vi "Dashboard Main.vi"() -> ()   [LabVIEW 2023]
uses:
  <vilib>/Utility/miscctls.llb/LVRectTypeDef.ctl
  <vilib>/event_ctls.llb/eventvkey.ctl
  <vilib>/Rock Robotics/WPI/DriverStation/WPI_DriverStationAllianceInfo.ctl
  b1c29fd4-b69e-4c47-bd92-218700034153.vi
  cd51690b-7cbe-44fb-a5f0-3232adb0ed53.vi
  a4e8d5d1-2ec3-4e81-be0b-60391cc68073.vi
  1b78be80-bab2-445d-a3e8-82f142a16380.vi
  9e807339-2903-4f51-8fcc-64b6a9381567.vi
  e75f20ac-3dfa-4544-8614-4803d6d17fbb.vi
  273c17a0-a238-4f2a-a55a-7e29d73850ff.vi
  87bdd142-1820-4e26-8582-f713a5f3da40.vi
  b8451b18-7b16-4e07-a196-a1bebf8ce026.vi
  5d307e9f-edd0-4132-a387-09c5916d43b1.vi
  0137daef-9682-45ba-80b9-2d4fda8852b8.vi
  f6a63fab-964b-4051-8314-d4414a0a258c.vi
  90e0fe9d-42b1-4a72-a6c8-4b9d9b3a5a2a.vi
  f15e925d-3118-43e3-bf67-a1272bbf81dd.vi
  394886aa-4cdd-4740-8681-89e3e438764a.vi
  77a42c1f-99bf-4bb6-8218-45b49017f7dc.vi
  5abae45b-ab2b-4816-ba0c-2a0b218f6531.vi
  31f70c1d-3051-4c77-9544-a691198ba614.vi
  f63f5451-5db6-487e-bc86-5cb81e92b132.vi
  81d0db6a-d68a-45c3-b3b1-458879412541.vi
  c235c188-eb56-46fb-93d3-e8acf396af31.vi
  115ba94a-0b26-47fa-ae73-5ec5bd9e502a.vi
  2422668c-951b-48e5-9bda-0f59c56d9c0d.vi
  7776664e-4af7-4b3d-b288-2266642a045e.vi
  6004ed5d-dfc4-4dad-95c1-8e371ea2b9cd.vi
  321ce103-7778-4bb1-9ecc-75a76fef05e9.vi
  d30e88cc-5e2b-4867-b271-53fc6d5cd4d7.vi
  fde90579-e212-4b8a-8145-a17c3e40bcbd.vi
  6c63589b-432e-4f9c-bacb-2063ed7bd576.vi
  b7dcf304-99f6-4f78-9d14-19aa8d9ea562.vi
  e8b3bb93-ba91-445b-94c6-9e998421f827.vi
  0480a820-69ef-45e6-a9f4-d7ff60c89e45.vi
  1c99237e-ea3d-4ecf-b7c2-61034db3ecd2.vi
  0a8fe2ab-d060-4915-a9b5-d8978247e2b6.vi
  b1c29fd4-b69e-4c47-bd92-218700034153.vi/77c742ae-e671-49bb-a825-a6e8cebc9f63.vi
  cd51690b-7cbe-44fb-a5f0-3232adb0ed53.vi/77c742ae-e671-49bb-a825-a6e8cebc9f63.vi
  a4e8d5d1-2ec3-4e81-be0b-60391cc68073.vi/77c742ae-e671-49bb-a825-a6e8cebc9f63.vi
  1b78be80-bab2-445d-a3e8-82f142a16380.vi/77c742ae-e671-49bb-a825-a6e8cebc9f63.vi
  9e807339-2903-4f51-8fcc-64b6a9381567.vi/77c742ae-e671-49bb-a825-a6e8cebc9f63.vi
  e75f20ac-3dfa-4544-8614-4803d6d17fbb.vi/77c742ae-e671-49bb-a825-a6e8cebc9f63.vi
  0137daef-9682-45ba-80b9-2d4fda8852b8.vi/77c742ae-e671-49bb-a825-a6e8cebc9f63.vi
  f6a63fab-964b-4051-8314-d4414a0a258c.vi/77c742ae-e671-49bb-a825-a6e8cebc9f63.vi
  90e0fe9d-42b1-4a72-a6c8-4b9d9b3a5a2a.vi/77c742ae-e671-49bb-a825-a6e8cebc9f63.vi
  f15e925d-3118-43e3-bf67-a1272bbf81dd.vi/77c742ae-e671-49bb-a825-a6e8cebc9f63.vi
  394886aa-4cdd-4740-8681-89e3e438764a.vi/77c742ae-e671-49bb-a825-a6e8cebc9f63.vi
  77a42c1f-99bf-4bb6-8218-45b49017f7dc.vi/77c742ae-e671-49bb-a825-a6e8cebc9f63.vi
  5abae45b-ab2b-4816-ba0c-2a0b218f6531.vi/77c742ae-e671-49bb-a825-a6e8cebc9f63.vi
  31f70c1d-3051-4c77-9544-a691198ba614.vi/77c742ae-e671-49bb-a825-a6e8cebc9f63.vi
  f63f5451-5db6-487e-bc86-5cb81e92b132.vi/77c742ae-e671-49bb-a825-a6e8cebc9f63.vi
  81d0db6a-d68a-45c3-b3b1-458879412541.vi/77c742ae-e671-49bb-a825-a6e8cebc9f63.vi
  c235c188-eb56-46fb-93d3-e8acf396af31.vi/77c742ae-e671-49bb-a825-a6e8cebc9f63.vi
  115ba94a-0b26-47fa-ae73-5ec5bd9e502a.vi/77c742ae-e671-49bb-a825-a6e8cebc9f63.vi
  2422668c-951b-48e5-9bda-0f59c56d9c0d.vi/77c742ae-e671-49bb-a825-a6e8cebc9f63.vi
  7776664e-4af7-4b3d-b288-2266642a045e.vi/77c742ae-e671-49bb-a825-a6e8cebc9f63.vi
  6004ed5d-dfc4-4dad-95c1-8e371ea2b9cd.vi/77c742ae-e671-49bb-a825-a6e8cebc9f63.vi
  321ce103-7778-4bb1-9ecc-75a76fef05e9.vi/77c742ae-e671-49bb-a825-a6e8cebc9f63.vi
  d30e88cc-5e2b-4867-b271-53fc6d5cd4d7.vi/77c742ae-e671-49bb-a825-a6e8cebc9f63.vi
  fde90579-e212-4b8a-8145-a17c3e40bcbd.vi/77c742ae-e671-49bb-a825-a6e8cebc9f63.vi
  6c63589b-432e-4f9c-bacb-2063ed7bd576.vi/77c742ae-e671-49bb-a825-a6e8cebc9f63.vi
  b7dcf304-99f6-4f78-9d14-19aa8d9ea562.vi/77c742ae-e671-49bb-a825-a6e8cebc9f63.vi
  e8b3bb93-ba91-445b-94c6-9e998421f827.vi/77c742ae-e671-49bb-a825-a6e8cebc9f63.vi
  0480a820-69ef-45e6-a9f4-d7ff60c89e45.vi/77c742ae-e671-49bb-a825-a6e8cebc9f63.vi
  1c99237e-ea3d-4ecf-b7c2-61034db3ecd2.vi/77c742ae-e671-49bb-a825-a6e8cebc9f63.vi
  0a8fe2ab-d060-4915-a9b5-d8978247e2b6.vi/77c742ae-e671-49bb-a825-a6e8cebc9f63.vi
  <vilib>/Utility/xml.llb/Read From XML File(array).vi
  <vilib>/Utility/xml.llb/Write to XML File(string).vi
  <vilib>/Rock Robotics/Network Tables/NT Read Number.vi
  <vilib>/Rock Robotics/Network Tables/NT Read Boolean.vi
  GlobalDashboard.vi
  <vilib>/Rock Robotics/Network Tables/NT Read String.vi
  <vilib>/Rock Robotics/Network Tables/NT Write Number.vi
  <vilib>/Rock Robotics/Network Tables/NT Read Numeric Array.vi
  <vilib>/Rock Robotics/Network Tables/NT Read String Array.vi
  <vilib>/Rock Robotics/Network Tables/NT Write Boolean.vi
  <vilib>/Rock Robotics/Network Tables/NT Read Boolean Array.vi
  <vilib>/Rock Robotics/Network Tables/NT Write String.vi
  <vilib>/Rock Robotics/Network Tables/NT Write Numeric Array.vi
  <vilib>/Rock Robotics/Network Tables/NT Write String Array.vi
  <vilib>/vision/NI_Vision_Development_Module.lvlib
panel:
  out "Indexer_Fault":bool
  out "Intake_Fault":bool
  out "Intake_Overheating":bool
  out "Elevator_Fault":bool
  out "Elevator_Overheating":bool
  in  "TCP":refnum<k5>
  in  "Dashboard Tab":T1(tab)=enum."Setup/Auto"
  in  "CheckList":i32(listbox)
  out "Heading_to_Target":dbl format="%.1f"
  out "Distance_to_Target":dbl format="%.1f"
  out "Robot_P":dbl format="%.1f"
  in  "Enable_Streaming_GUI":bool=TRUE
  out "Robot_Profile_GUI":string
  out "Auto_Playbook_GUI":string
  in  "Select Driver Profile":u16(ring) items=["N/A"]
  in  "Camera Name":string(combo)="limelight"
  in  "Camera Settings":T2={"Frame Rate"=20, "Compression"=60, "Size"=1, "DB Camera Config"=FALSE} {"Size" items=["640x480", "320x240", "160x120"]}
  in  "Select Autonomous Play":u16(ring) items=["N/A"]
  out "Master_Caution_GUI_0":bool caption="Mode_Butterfly"
  out "Robot_is_Autonomous_GUI_0":bool caption="Mode_Butterfly"
  out "Robot_Code_Version_GUI":string
  out "Auto_Suffix_GUI":string
  in  "Refresh_Auto_Play_List_GUI":bool
  in  "Auto_Delay_GUI":dbl format="%.1f"
  in  "Manual_Start_X":dbl min=0.0 max=700.0 format="%.1f"
  out "Robot_X":dbl format="%.1f"
  out "Robot_Y":dbl format="%.1f"
  in  "Manual_Start_Y":dbl min=0.0 max=400.0 format="%.1f"
  out "Robot_H_GUI":dbl format="%.1f"
  in  "Manual_Start_H":dbl min=0.0 max=360.0 format="%.1f"
  in  "Field Map":u16(ring) items=["N/A"]
  in  "Push_Robot_Start_GUI":bool
  in  "Export_Robot_Pose":bool
  in  "Clear_Robot_Pose_Display":bool
  in  "Dock_Dashboard":bool
  in  "Force_Human_Control_GUI":bool
  in  "Auto_Test_Mode_GUI":bool
  in  "Disable_Fusion_While_Autonomous":bool
  in  "Disable_Fusion_While_Disabled":bool=TRUE
  out "Robot Pose 1":cluster{dbl[], dbl[]}[](graph)
  out "Master_State_TRAP_Indicator":bool
  out "Master_State_CLIMB_Indicator":bool
  out "Master_State_AMP_Indicator":bool
  out "Help Graphic":T3(plugin-control)
  out "LL_Ret_Left":bool
  out "LL_Ret_Right":bool
  out "WA_Ret_Right":bool
  out "WA_Ret_Left":bool
  out "Swerve_Drive_Fault":bool
  out "State_Score":bool
  out "State_Shelf":bool
  out "Robot Pose 2":cluster{dbl[], dbl[]}[](graph)
  out "Master_State_SPEAKER_Indicator":bool
  out "Vision_Fault_GUI":bool
  out "Pressure_Leak_GUI":bool
  in  "Master_Safety_Override_1":bool
  in  "Manipulator_Help":bool
  in  "Driver_Help":bool
  out "No_Secondary_Camera":bool
  out "Swerve_Shifter_Failure":bool
  out "Electrical_Fault_GUI":bool
  out "Diverting_Power_GUI":bool
  out "CAN_Bus_Fault_GUI":bool
  out "IMU_Failure_GUI":bool
  out "Robot_is_Autonomous_GUI_1":bool caption="Mode_Butterfly"
  out "LL_Valid":bool caption="Mode_Butterfly"
  out "Auto_Error_GUI":bool
  in  "Clear_Errors_GUI":bool
  out "Swerve_Azimuth_Fault":bool
  out "Pressure_Transducer_GUI":dbl(slide) scale=0.0..115.0
  out "Pressure_Vent_GUI":bool
  out "Swerve_Overheating":bool
  out "Compressor_On_GUI":bool
  in  "Right":bool
  in  "Reticule":T4(ring)
  in  "Save":bool
  in  "Up":bool
  in  "Down":bool
  in  "Left":bool
  out "Master_Caution_GUI_1":bool caption="Mode_Butterfly"
  out "Battery_Critical_GUI":bool
  out "Battery_Voltage_GUI":dbl(slide) scale=11.0..13.0
  out "Field_Oriented_GUI":bool caption="Mode_Butterfly"
  out "Slow_Loop":bool
  out "Combined Camera Feed":T3(plugin-control)
  in  "Camera_Override_GUI":bool
  in  "Field_Oriented_Override_GUI":bool
  out "Pointed_at_Target":bool caption="Mode_Butterfly"
  in  "Auto_Targeting_Override":bool
  out "State_Hopper":bool
  out "Using_Auto_Targeting":bool caption="Mode_Butterfly"
  out "Swerve_Output_Loop_Time_GU":u32
  out "Swerve_3_Drive_Velocity":dbl format="%.1f"
  out "Swerve_3_Azimuth_Position":dbl format="%.1f"
  out "Swerve_3_Drive_Temperature":dbl
  out "Swerve_0_Drive_Temperature":dbl
  out "Camera Perf":string
  out "Control_Loop_Time_GUI":u32
  in  "Calibrate_Wheels_GUI":bool
  in  "Home_Wheels_GUI":bool
  out "Swerve_0_Azimuth_Position":dbl format="%.1f"
  out "Swerve_0_Drive_Velocity":dbl format="%.1f"
  out "Swerve_1_Drive_Velocity":dbl format="%.1f"
  out "Swerve_1_Azimuth_Position":dbl format="%.1f"
  out "Swerve_1_Drive_Temperature":dbl
  out "Swerve_2_Drive_Velocity":dbl format="%.1f"
  out "Swerve_2_Azimuth_Position":dbl format="%.1f"
  out "Swerve_2_Drive_Temperature":dbl
  in  "Arm_Calibrate_Wheels_GUI":bool
  out "Master_Caution_GUI_2":bool caption="Mode_Butterfly"
  in  "Actuator Testing":u16(ring) items=["N/A"]
  in  "Test_Actuator_Value_GUI":dbl step=0.1 format="%.2f"
  in  "Calibrate_Joysticks_GUI":bool
  in  "Arm_Calibrate_Joysticks":bool
  out "Robot_is_Autonomous_GUI_2":bool caption="Mode_Butterfly"
  in  "Test_Actuator_Period_GUI":dbl min=0.0 step=1.0 format="%.2f"
  out "Pose_Loop_Time_GUI":u32
  in  "Mute_Audible_Warnings":bool
  out "Combined Error String":string
  out "Swerve_0_Shifter_State":string
  out "Swerve_1_Shifter_State":string
  out "Swerve_3_Shifter_State":string
  out "Swerve_2_Shifter_State":string
  out "Swerve_Azimuth_Fault_Array":bool[](array[boolean])
  in  "Super_Test_Mode_GUI":bool
  out "Current_Driver_Profile_Setpoints_GUI":T5={"Strafe Deadband"=0.08, "Strafe Scaling"=2.0, "Strafe Maximum"=0.5, "Rotation Deadband"=0.15, "Rotation Scaling"=2.5, "Rotation Maximum"=0.5} {"Rotation Maximum" min=0.3 max=1.0 scale=0.3..1.0; "Rotation Scaling" min=1.0 max=4.0 scale=1.0..4.0; "Rotation Deadband" min=0.0 max=0.25 scale=0.0..0.25; "Strafe Maximum" min=0.3 max=1.0 scale=0.3..1.0; "Strafe Scaling" min=1.0 max=4.0 scale=1.0..4.0; "Strafe Deadband" min=0.0 max=0.25 scale=0.0..0.25}
  in  "New_Driver_Profile_Setpoints_GUI":T6={"Strafe Deadband"=0.08, "Strafe Scaling"=2.0, "Strafe Max"=0.5, "Rotate Deadband"=0.15, "Rotate Scaling"=2.5, "Rotate Max"=0.5} {"Rotate Max" min=0.3 max=1.0 format="%.2g"; "Rotate Scaling" min=1.0 max=4.0 format="%.2g"; "Rotate Deadband" min=0.0 max=0.25 format="%.2g"; "Strafe Max" min=0.3 max=1.0 format="%.2g"; "Strafe Scaling" min=1.0 max=4.0 format="%.2g"; "Strafe Deadband" min=0.0 max=0.25 format="%.2g"}
  in  "Apply_Driver_Profile_Setpoints_GUI":bool
  out "Current_Driver_Profile_GUI":string
  in  "Free_Tuning_Variable_GUI":dbl min=0.0 step=1.0 format="%.3f"
  out "Audible_Warnings_Enabled_GUI":bool
  out "Legal_Drivers_GUI":string[](array[string])
  out "Swerve_Shifter_Failure_Array":bool[](array[boolean])
  out "Swerve_Overheating_Array":bool[](array[boolean])
  out "Swerve_Drive_Fault_Array":bool[](array[boolean])
  out "NT Connection":bool
  out "Mode":T7(ring)=enum."Auto Disabled"
  out "Tree":string(tree)
  out "Background":bool
  # "2023 Dashboard v2.3-stable"
  # "Robot Profile"
  # "Robot X Position (in)"
  # "Robot Y Position (in)"
  # "Delay (s)"
  # "Robot Heading (deg)"
  # "Suffix"
  # "X (in)"
  # "Robot Pitch (deg)"
  # "Autonomous Playbook Entry"
  # "Auto Test\nMode"
  # "Force\nHuman"
  # "Y (in)"
  # "Target Distance (in)"
  # "Target Heading (deg)"
  # "H (deg)"
  # "Undock Dashboard"
  # "Yes Camera Streaming"
  # "Stop Fusion While Auto"
  # "Stop Fusion While Disabled"
  # "X"
  # "Y"
  # "MASTER\nSTATES"
  # "OVERRIDES"
  # "Camera Override"
  # "Robot-Oriented Drive Controls"
  # "Auto-Targeting Override"
  # "Disengage\nSafeties"
  # "11"
  # "13"
  # "0"
  # "120"
  # "Drivebase Subsytem"
  # "Driver Profile Selected"
  # "Loop Times"
  # "Module 1"
  # "Module 0"
  # "Control (ms)"
  # "Azimuth (deg)"
  # "Pose (ms)"
  # "Temp (C)"
  # "Drive Output (ms)"
  # "Velocity (ft/s)"
  # "Shifter State"
  # "Module 2"
  # "Module 3"
  # "Variable (bleh)"
  # "Disabled\nTest Mode"
  # "Azimuth (deg)"
  # "Temp (C)"
  # "Velocity (ft/s)"
  # "Shifter State"
  # "Calibrate Wheels"
  # "Period (s)"
  # "Calibrate Joysticks"
  # "Amplitude"
  # "0"
  # "0.25"
  # "1"
  # "4"
  # "0.3"
  # "1"
  # "0"
  # "0.25"
  # "1"
  # "4"
  # "0.3"
  # "1"
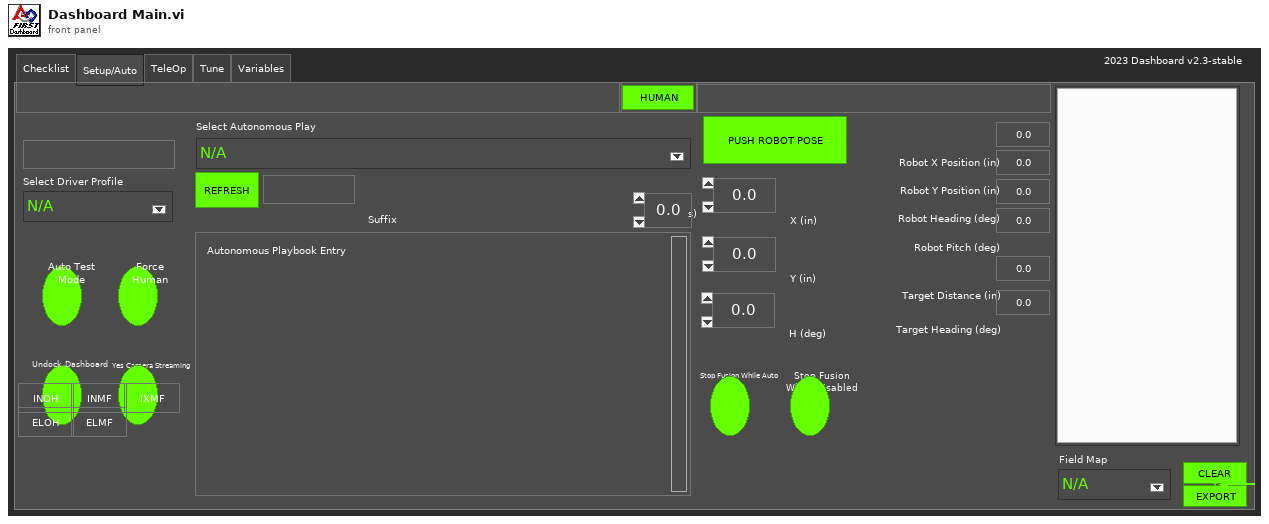
[diagram p1: front panel]
types:
  T1 = enum32{"Checklist", "Setup/Auto", "TeleOp", "Tune", "NT", "Test", "Commands", "Variables"}
  T2 = cluster{"Frame Rate":i32, "Compression":i32, "Size":u16, "DB Camera Config":bool}
  T3 = typedef "IMAQ Image.ctl" = refnum<image>
  T4 = enum16{"Wide Angle Left Reticule", "Wide Angle Right Reticule", "Lime Light Left Reticule", "Lime Light Right Reticule"}
  T5 = cluster{"Strafe Deadband":dbl, "Strafe Scaling":dbl, "Strafe Maximum":dbl, "Rotation Deadband":dbl, "Rotation Scaling":dbl, "Rotation Maximum":dbl}
  T6 = cluster{"Strafe Deadband":dbl, "Strafe Scaling":dbl, "Strafe Max":dbl, "Rotate Deadband":dbl, "Rotate Scaling":dbl, "Rotate Max":dbl}
  T7 = enum8{"Tele-Op Disabled", "Tele-Op Enabled", "Auto Disabled", "Auto Enabled", "Test Disabled", "Test Enabled", "Disconnected", "No Code", "E-Stop"}
  T8 = cluster{"Save Path":path, "Interval (s)":dbl, "Keep":i32}
  T9 = enum32{"Drive", "Camera", "Basic", "Custom", "Test", "Commands", "Checklist", "Variables"}
  T10 = cluster{"IDs":cluster{"RPC field ID":u16, "Unique ID":u16}, "String":string}
  T11 = typedef "Image Type" = u32
  T12 = typedef "WPI_DriverStationAllianceInfo.ctl" = enum16{"Red", "Blue", "Invalid"}
  T13 = enum8{"Enabled", "Disabled", "Disabled and Grayed Out"}
  T14 = cluster{"Error Strings":string, "Disable Counts":cluster{u16, u16}, "Rail Faults":cluster{u16, u16, u16}, "Robot IP":string, "DB Mode":u8, "Event Info":cluster{"Name":string, "Type":u8, "Number":u16, "Replay":u8}}
  T15 = cluster{"Storage":cluster{"Disk Free":u64, "RAM Block":u32, "RAM free":u32}, "CPU Utilization":cluster{"CPU % ISR":sgl, "CPU % Time Crit":sgl, "CPU % Timed Str":sgl, "CPU % High":sgl, "CPU % Above":sgl, "CPU % Normal":sgl, "CPU % Low":sgl}, "CAN":cluster{"% Bus Utilization":sgl, "Bus Off Cnt":u32, "TX_FIFO Full Cnt":u32, "Receive Error Cnt":u8, "Transmit Error Cnt":u8}, "HID":cluster{"HID Outputs":u32, "Rumble Low":u16, "Rumble High":u16}[]}
  T16 = cluster{"Status bits":cluster{"Test Mode":bool, "Autonomous":bool, "Enabled":bool, "Code Start":bool, "Brownout":bool, "Reserved 2":bool, "Reserved 3":bool, "E-Stop":bool}, "Code Trace":cluster{"Disabled":bool, "TeleOp":bool, "Auto":bool, "Test":bool}, "Controller Type":enum16{"unknown", "cRIO", "roboRio"}, "Code?":enum16{"unknown", "noCode", "code"}, "Battery V":dbl}
  T17 = cluster{"Control Bits":cluster{"TestMode":bool, "Autonomous":bool, "Enabled":bool, "FMS Present":bool, bool, bool, bool, "E-Stop":bool}, "Team Station ":u8, "Countdown":sgl, "Joystick Values":cluster{"Axes":dbl[], "Buttons":bool[], "POVs":i16[]}[]}
  T18 = typedef "imagedata.ctl" = cluster{"image type":i32, "image depth":i32, "image":u8[], "mask":u8[], "colors":u32[], "Rectangle":cluster{"left":i16, "top":i16, "right":i16, "bottom":i16}}
  T19 = cluster{"Boolean":bool, "Numeric Text.Text Colors:Text Color":u32}
  T20 = cluster{"value[0]":dbl, "value[1]":dbl, "value[2]":dbl, "value[3]":dbl, "value[4]":dbl, "value[5]":dbl}
  T21 = typedef "LVRectTypeDef.ctl" = cluster{"Left":i16, "Top":i16, "Right":i16, "Bottom":i16}
  T22 = typedef "eventvkey.ctl" = enum16{"ASCII", "Enter", "Return", "Shift", "Ctrl", "Alt", "Cmd", "Opt", "Caps", "NumLock", "Clear", "Break", "Up", "Down", "Left", "Right", "Insert", "Delete", "Home", "End", "PageUp", "PageDown", "Escape", "Help", "Pause", "ScrollLock", "F1", "F2", "F3", "F4", "F5", "F6", "F7", "F8", "F9", "F10", "F11", "F12", "F13", "F14", "F15", "F16", "F17", "F18", "F19", "F20", "F21", "F22", "F23", "F24", "Play", "VolumeUp", "VolumeDown", "Mute", "Two Byte Char"}
  T23 = cluster{"Shift":bool, "Ctrl":bool, "Alt":bool, "Cmd":bool, "Opt":bool}
  T24 = cluster{"WA_Ret_Left":refnum<vi>, "WA_Ret_Right":refnum<vi>, "LL_Ret_Left":refnum<vi>, "LL_Ret_Right":refnum<vi>}
  T25 = cluster{"Camera Name":string, string, "Saved DB Images Info":cluster{"Save Path":path, "Interval (s)":dbl, "Keep":i32}}
  T26 = cluster{string, "Swerve_Shifter_Failure":bool, dbl}
  T27 = cluster{string, "Master_Safety_Override_1":bool, dbl}
  T28 = cluster{string, "Swerve_Azimuth_Fault":bool, dbl}
  T29 = cluster{string, "Arm_Calibrate_Wheels_GUI":bool, dbl}
  T30 = cluster{string, "Electrical_Fault_GUI":bool, dbl}
  T31 = cluster{string, "Arm_Calibrate_Joysticks":bool, dbl}
  T32 = cluster{string, "Swerve_Drive_Fault":bool, dbl}[]
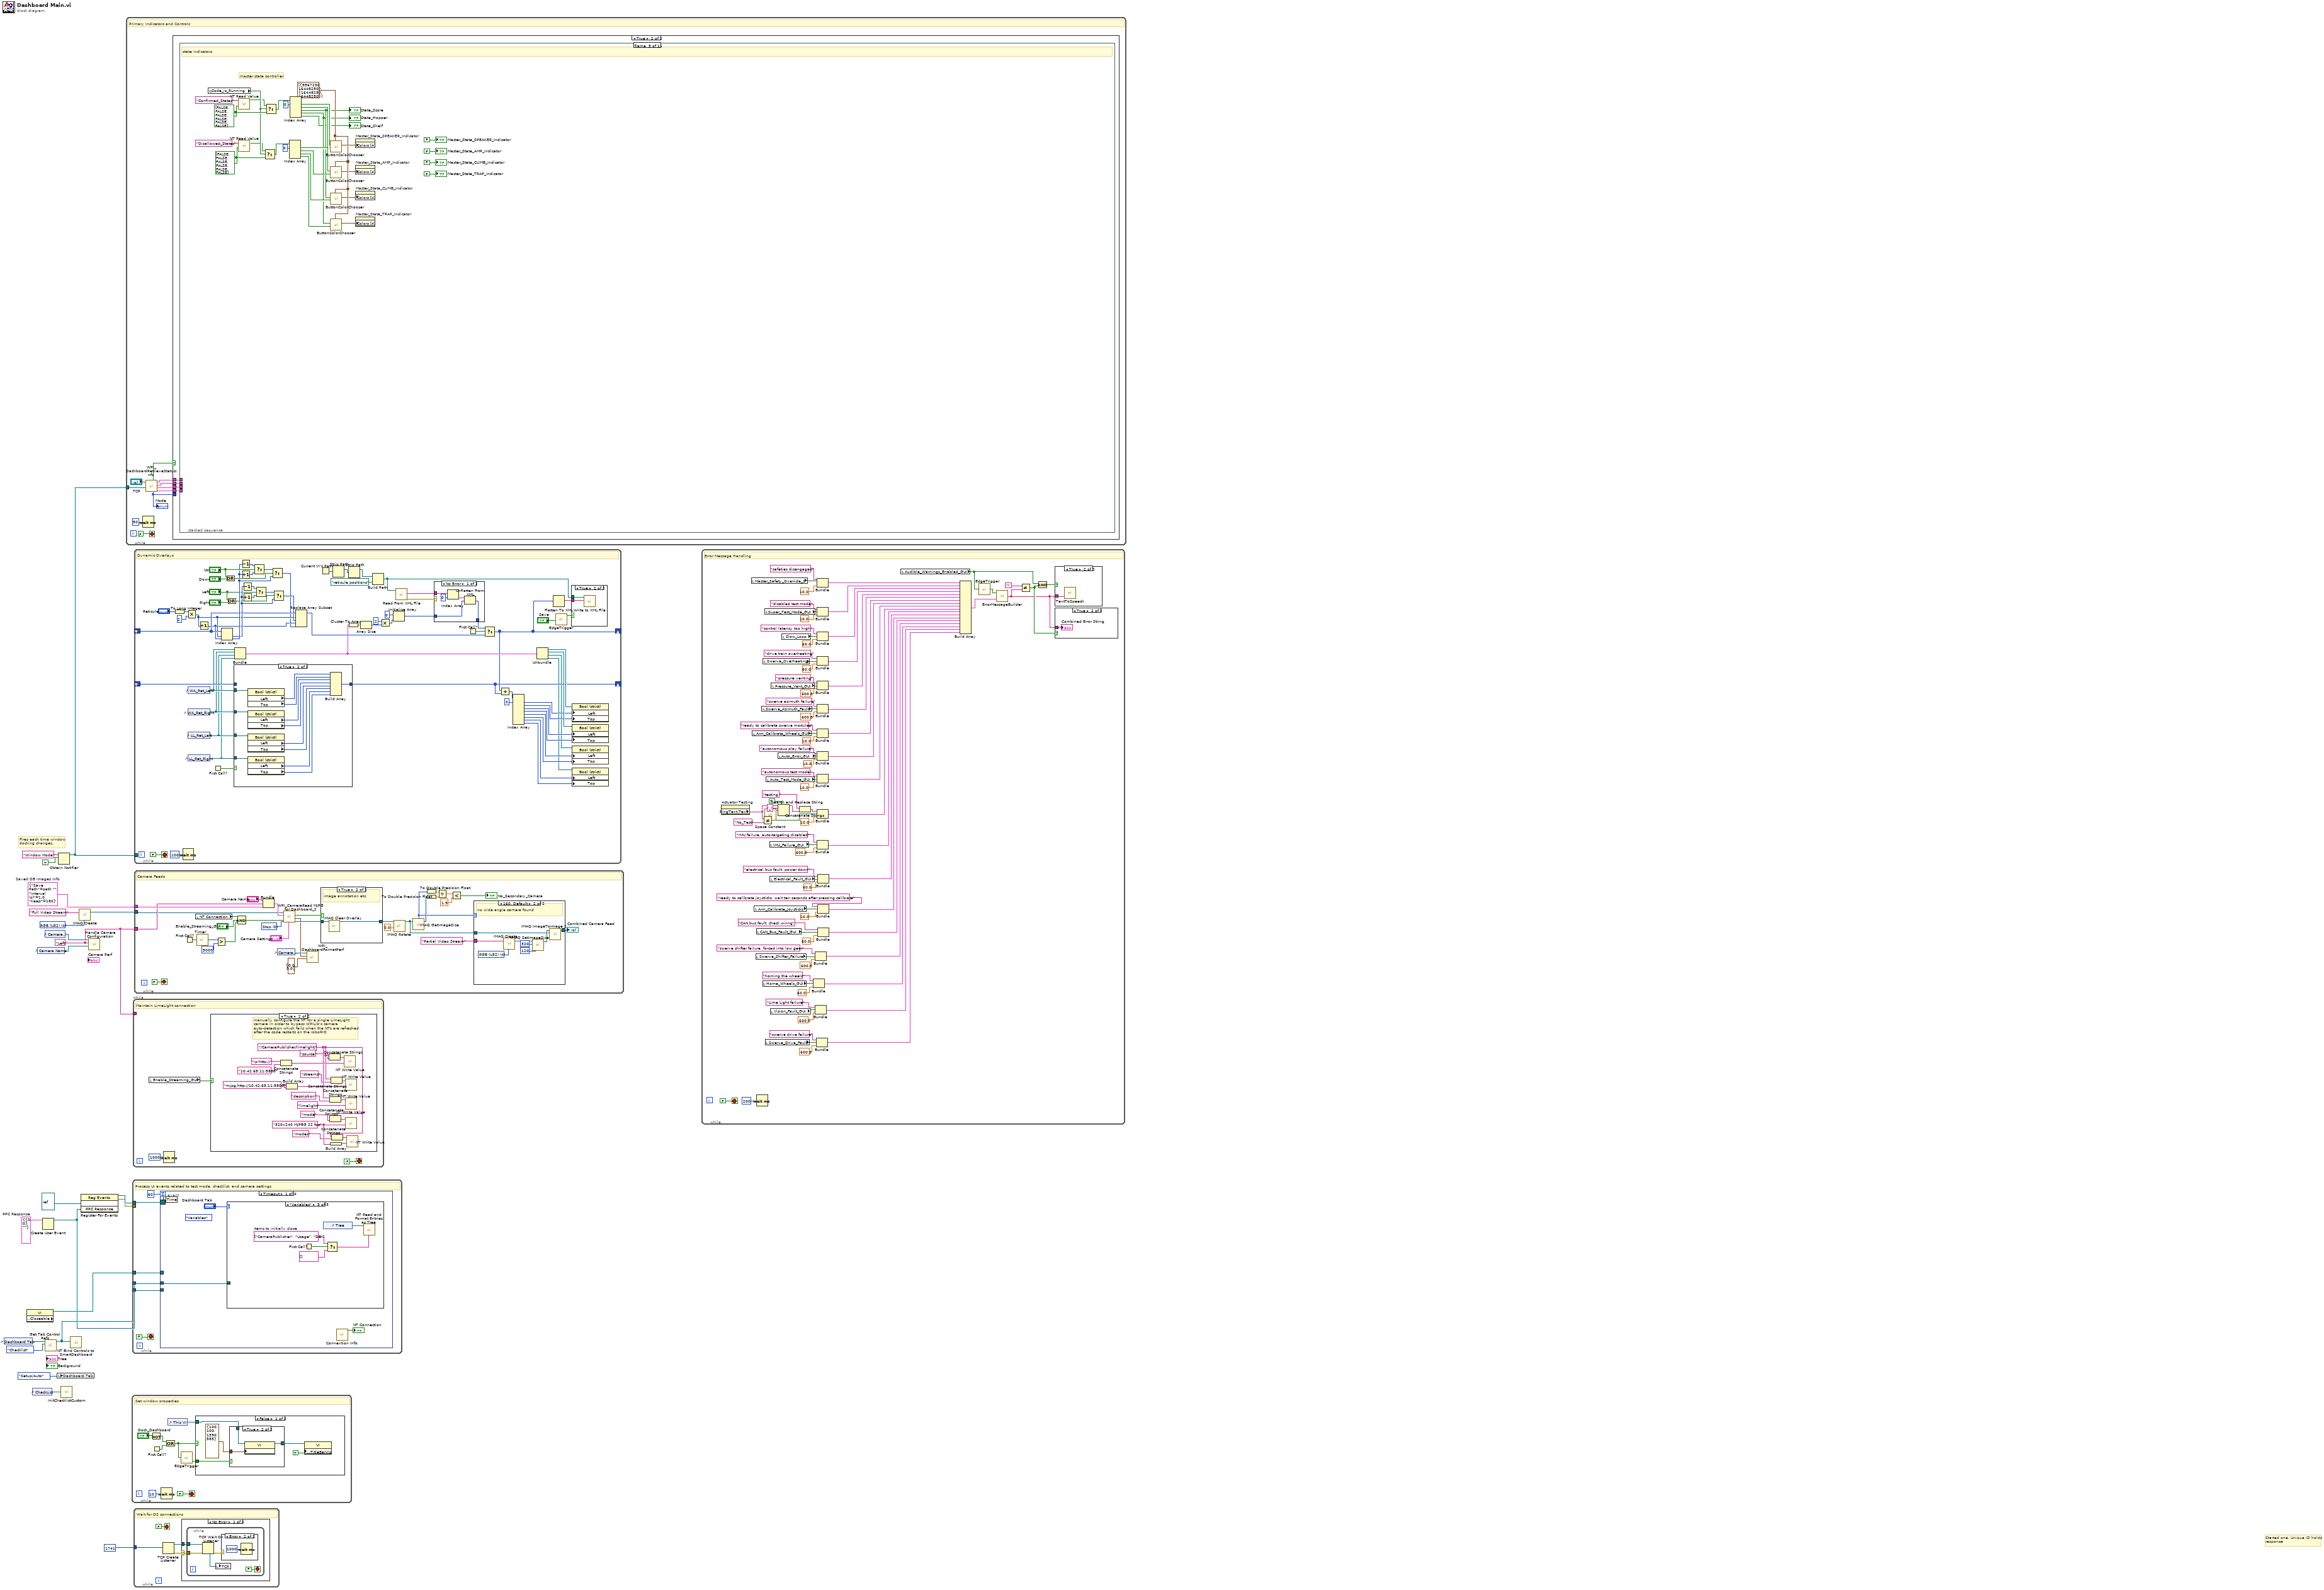
[diagram p0: block diagram]
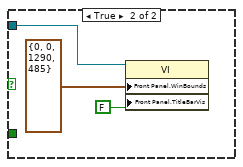
[diagram p4: hidden frame]
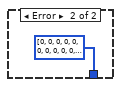
[diagram p7: hidden frame]
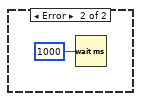
[diagram p11: hidden frame]
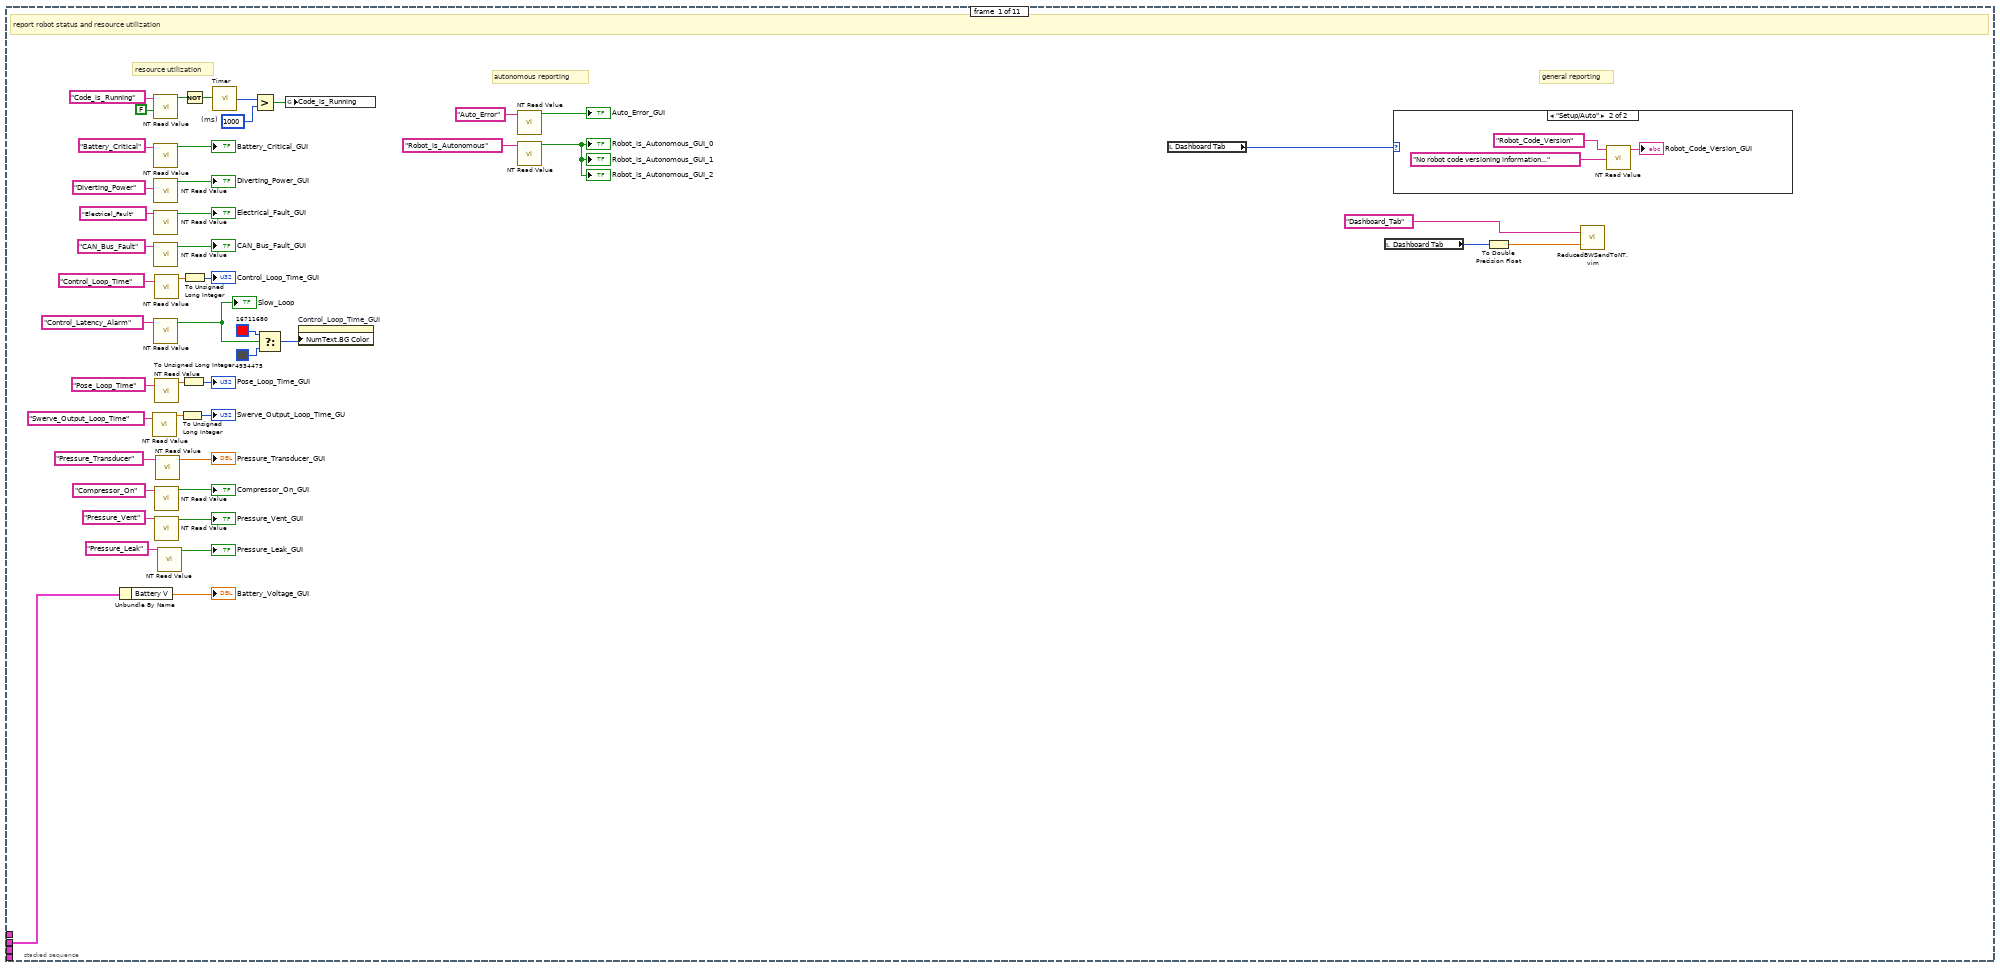
[diagram p13: hidden frame]
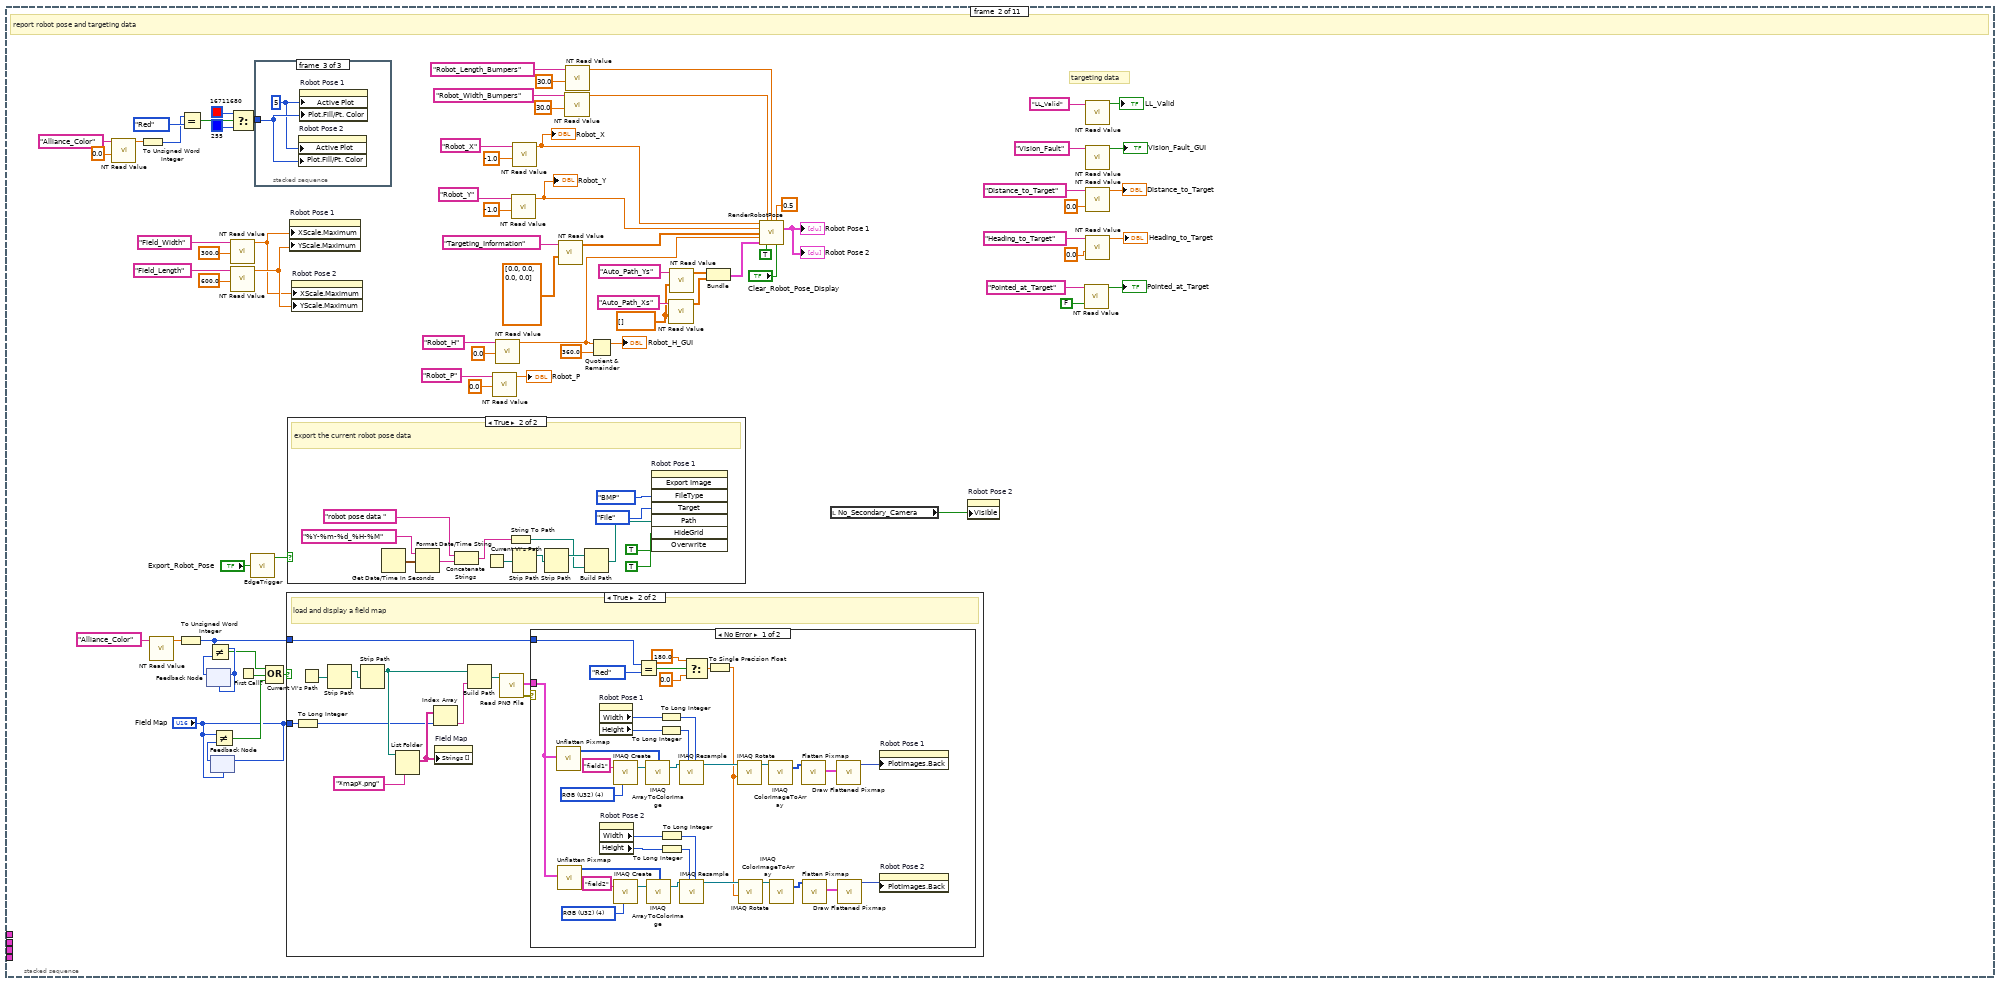
[diagram p15: hidden frame]
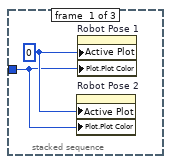
[diagram p16: hidden frame]
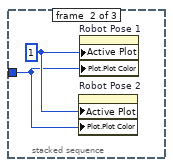
[diagram p17: hidden frame]
diagram:
  w10 = T8 {"Save Path"=path "", "Interval (s)"=1.0, "Keep"=180}  # Saved DB Images Info
  w3 = "Left"
  w13 = T10 {"IDs"={"RPC field ID"=0, "Unique ID"=0}, "String"=""}  # RPC Response
  w6 = T11 4 items=["Grayscale (U8)", "Grayscale (I16)", "Grayscale (SGL)", "Complex (CSG)", "RGB (U32)", "HSL (U32)", "RGB (U64)"] ("Image Type")
  # "Started one, Unique ID holds\nresponse"
  # "Fires each time window\ndocking changes."
  n1 = control-ref of="Dashboard Tab"() -> (w16:refnum<vi>)
  n2 = property class="VI" props=["Front Panel.Closeable"]() -> (reference out=w17:refnum<vi>)  [unwired: 2 in, 2 out]
  n3 = control-ref of="CheckList"() -> (w5:refnum<vi>)
  n4 = control-ref of="Camera Name"() -> (w8:refnum<vi>)
  n5 = Create User Event(user event datatype=w13) -> (user event=w12:refnum<user-event>)  [unwired: 1 in, 1 out]
  n6 = control-ref of="Camera Settings"() -> (w9:refnum<vi>)
  n7 = call <vilib>:"Get Tab Control Refs.vi"("Page Index"=T9."Checklist" ("Dashboard Tab"), "TabControl in"=w16) -> ("ControlsOnPage"=w2:refnum<vi>[])  [unwired: 9 in]
  n8 = local write "Dashboard Tab"(T1."Setup/Auto" ("Dashboard Tab")) -> ()
  n9 = Obtain Notifier(name (unnamed)="Window Mode", notification data type=TRUE) -> (notifier out=w1:refnum<notifier>)  [unwired: 2 in, 2 out]
  n10 = call "InitChecklistCustom.vi"("ListBox in"=w5) -> ()  [unwired: 1 in]
  n11 = call <vilib>:"NT Bind Controls to SmartDashboard.vi"("Bound Control Refs"=w2) -> ()  [unwired: 11 in]
  n12 = call "IMAQ Create"("Image Name"="Full Video Stream", "Image Type"=w6) -> ("New Image"=w4:T3)  [unwired: 2 in, 2 out]
  n13 = register-events(refnum<vi> refnum, w12) -> (reference out=w20:refnum<event-registration>, error out=w19:errorcluster)  [unwired: 2 in]
  n14 = call "Handle Camera Configuration.vi"("CameraNameRef"=w8, "Display Name"=w3, "ClusterRef"=w9) -> ()  [unwired: 9 in]
  n15 = while {
    tunnel: w1 -> [w24]
    stop <- FALSE stop-if-true
    # "Primary Indicators and Controls"
    n16 = Wait (ms)(milliseconds to wait=u32 50) -> ()  [unwired: 1 out]
    n17 = call <vilib>:"WPI_DashboardRetrieveStatusInfo.vi"("Window Mode Notifier"=w24, "TCP Cnx"="TCP") -> ("Power and Errors"=w27:T14, "Robot Metrics"=w30:T15, "Status Info"=w31:T16, "Control Info"=w28:T17, "Robot Mode"=w26:T7, "Process?"=w29:bool)  [unwired: 4 in]
    "Mode" <- w26
    n18 = case shown="True" w29 {
      tunnel: w31 -> [_ w35]
      tunnel: w30 -> [_ w34]
      tunnel: w28 -> [_ w36]
      tunnel: w27 -> [_ w33]
      tunnel: w26 -> [_ _]
      frame False {
      }
      frame True {
        n19 = stacked-sequence {
          tunnel: w36 -> [_ _ _ _ _ _ _ _ _ _ _]
          tunnel: w35 -> [w51 _ _ _ _ _ _ _ _ _ _]
          tunnel: w34 -> [_ _ _ _ _ _ _ _ _ _ _]
          tunnel: w33 -> [_ _ _ _ _ _ _ _ _ _ _]
          frame #0 {
            w41 = u32 1000  # (ms)
            # "general reporting"
            # "resource utilization"
            # "autonomous reporting"
            # "report robot status and resource utilization"
            n20 = Unbundle By Name(w51) -> ("Battery V"=→"Battery_Voltage_GUI":dbl)
            n21 = call-poly <vilib>:"NT Read Value.vi"("name"="Swerve_Output_Loop_Time" ("Name")) -> ("value"=w39:dbl)  [unwired: 8 in, 2 out]
            n22 = call-poly <vilib>:"NT Read Value.vi"("default value"=FALSE, "name"="Code_is_Running" ("Name")) -> ("value"=w44:bool)  [unwired: 7 in, 2 out]
            n23 = call-poly <vilib>:"NT Read Value.vi"("name"="Battery_Critical" ("Name")) -> ("value"=→"Battery_Critical_GUI":bool)  [unwired: 8 in, 2 out]
            n24 = call-poly <vilib>:"NT Read Value.vi"("name"="Diverting_Power" ("Name")) -> ("value"=→"Diverting_Power_GUI":bool)  [unwired: 8 in, 2 out]
            n25 = call-poly <vilib>:"NT Read Value.vi"("name"="Electrical_Fault" ("Name")) -> ("value"=→"Electrical_Fault_GUI":bool)  [unwired: 8 in, 2 out]
            n26 = call-poly <vilib>:"NT Read Value.vi"("name"="CAN_Bus_Fault" ("Name")) -> ("value"=→"CAN_Bus_Fault_GUI":bool)  [unwired: 8 in, 2 out]
            n27 = call-poly <vilib>:"NT Read Value.vi"("name"="Control_Latency_Alarm" ("Name")) -> ("value"=w80:bool)  [unwired: 8 in, 2 out]
            "Slow_Loop" <- w80
            n28 = call-poly <vilib>:"NT Read Value.vi"("name"="Control_Loop_Time" ("Name")) -> ("value"=w71:dbl)  [unwired: 8 in, 2 out]
            n29 = call-poly <vilib>:"NT Read Value.vi"("name"="Pose_Loop_Time" ("Name")) -> ("value"=w81:dbl)  [unwired: 8 in, 2 out]
            n30 = call-poly <vilib>:"NT Read Value.vi"("name"="Compressor_On" ("Name")) -> ("value"=→"Compressor_On_GUI":bool)  [unwired: 8 in, 2 out]
            n31 = call-poly <vilib>:"NT Read Value.vi"("name"="Pressure_Vent" ("Name")) -> ("value"=→"Pressure_Vent_GUI":bool)  [unwired: 8 in, 2 out]
            n32 = call-poly <vilib>:"NT Read Value.vi"("name"="Pressure_Transducer" ("Name")) -> ("value"=→"Pressure_Transducer_GUI":dbl)  [unwired: 8 in, 2 out]
            n33 = call-poly <vilib>:"NT Read Value.vi"("name"="Pressure_Leak" ("Name")) -> ("value"=→"Pressure_Leak_GUI":bool)  [unwired: 8 in, 2 out]
            n34 = To Unsigned Long Integer(number=w39) -> (unsigned 32bit integer=→"Swerve_Output_Loop_Time_GU":u32)
            n35 = To Unsigned Long Integer(number=w81) -> (unsigned 32bit integer=→"Pose_Loop_Time_GUI":u32)
            n36 = Not(x=w44) -> (.not. x?=w43:bool)
            n37 = To Unsigned Long Integer(number=w71) -> (unsigned 32bit integer=→"Control_Loop_Time_GUI":u32)
            n38 = call "Timer.vi"("Reset Timer"=w43) -> ("Time (ms)"=w42:u32)
            n39 = Greater?(x=w42, y=w41) -> (0:w40:bool)
            n40 = Select(t=u32 16711680 ("Numeric Text.Text Colors:Text Color"), s=w80, f=u32 4934475 ("Numeric Text.Text Colors:Text Color")) -> (s? t:f=w75:u32)
            n41 = global write "GlobalDashboard.vi" "Code_is_Running"(w40) -> ()
            n42 = property on="Control_Loop_Time_GUI" class="DigNum (strict)"("NumText.BG Color"=w75) -> ()  [unwired: 2 in, 2 out]
            n43 = call-poly <vilib>:"NT Read Value.vi"("name"="Auto_Error" ("Name")) -> ("value"=→"Auto_Error_GUI":bool)  [unwired: 8 in, 2 out]
            n44 = call-poly <vilib>:"NT Read Value.vi"("name"="Robot_is_Autonomous" ("Name")) -> ("value"=→"Robot_is_Autonomous_GUI_0" →"Robot_is_Autonomous_GUI_1" →"Robot_is_Autonomous_GUI_2":bool)  [unwired: 8 in, 2 out]
            n45 = local read "Dashboard Tab"() -> (w47:T1)
            n46 = local read "Dashboard Tab"() -> (w48:T1)
            n47 = case shown="\"Setup/Auto\"" w47 {
              frame "Checklist", Default {
              }
              frame "Setup/Auto" {
                n48 = call-poly <vilib>:"NT Read Value.vi"("default value"="No robot code versioning information..." ("Default Value"), "name"="Robot_Code_Version" ("Name")) -> ("value"=→"Robot_Code_Version_GUI":string)  [unwired: 7 in, 2 out]
              }
            }
            n49 = To Double Precision Float(number=w48) -> (double precision float=w49:dbl)
            n50 = call "ReducedBWSendToNT.vim"("Value In"=w49, "NT Name"="Dashboard_Tab" ("Name")) -> ()  [unwired: 1 out]
          }
          frame #1 {
            w87 = dbl[] [] ("default value")
            # "targeting data"
            # "report robot pose and targeting data"
            n51 = call-poly <vilib>:"NT Read Value.vi"("default value"=0.0, "name"="Alliance_Color" ("Name")) -> ("value"=w117:dbl)  [unwired: 7 in, 2 out]
            n52 = To Unsigned Word Integer(number=w117) -> (unsigned 16bit integer=w115:u16)
            n53 = call-poly <vilib>:"NT Read Value.vi"("name"="Alliance_Color" ("Name")) -> ("value"=w135:dbl)  [unwired: 8 in, 2 out]
            n54 = To Unsigned Word Integer(number=w135) -> (unsigned 16bit integer=w145:u16)
            n55 = Equal?(x=w115, y=WPI_DriverStationAllianceInfo."Red" ("x")) -> (x = y?=w108:bool)
            n56 = feedback #1(w145) -> (w141:u16)
            n57 = feedback-in #1(w145) -> ()
            n58 = Not Equal?(x=w145, y=w141) -> (x != y?=w143:bool)
            n59 = feedback #2("Field Map") -> (w146:u16)
            n60 = feedback-in #2("Field Map") -> ()
            n61 = Not Equal?(x="Field Map", y=w146) -> (x != y?=w148:bool)
            n62 = call-poly <vilib>:"NT Read Value.vi"("default value"=300.0 ("Default Value"), "name"="Field_Width" ("Name")) -> ("value"=w109:dbl)  [unwired: 7 in, 2 out]
            n63 = call-poly <vilib>:"NT Read Value.vi"("default value"=600.0 ("Default Value"), "name"="Field_Length" ("Name")) -> ("value"=w110:dbl)  [unwired: 7 in, 2 out]
            n64 = Select(t=u32 16711680 ("Color"), s=w108, f=u32 255 ("Color")) -> (s? t:f=w111:u32)
            n65 = First Call?() -> (First Call?: T/F=w142:bool)
            n66 = call "EdgeTrigger.vi"("Input Signal"="Export_Robot_Pose") -> ("Rising Edge Trigger"=w149:bool)  [unwired: 2 out]
            n67 = stacked-sequence {
              tunnel: w111 -> [w161 w163 w166]
              frame #0 {
                w162 = u32 0 ("Active Plot")
                n68 = property on="Robot Pose 2" class="XYGraph (strict)"("Active Plot"=w162, "Plot.Plot Color"=w161) -> ()  [unwired: 2 in, 2 out]
                n69 = property on="Robot Pose 1" class="XYGraph (strict)"("Active Plot"=w162, "Plot.Plot Color"=w161) -> ()  [unwired: 2 in, 2 out]
              }
              frame #1 {
                w164 = u32 1 ("Active Plot")
                n70 = property on="Robot Pose 2" class="XYGraph (strict)"("Active Plot"=w164, "Plot.Plot Color"=w163) -> ()  [unwired: 2 in, 2 out]
                n71 = property on="Robot Pose 1" class="XYGraph (strict)"("Active Plot"=w164, "Plot.Plot Color"=w163) -> ()  [unwired: 2 in, 2 out]
              }
              frame #2 {
                w165 = u32 5 ("Active Plot")
                n72 = property on="Robot Pose 2" class="XYGraph (strict)"("Active Plot"=w165, "Plot.Fill/Pt. Color"=w166) -> ()  [unwired: 2 in, 2 out]
                n73 = property on="Robot Pose 1" class="XYGraph (strict)"("Active Plot"=w165, "Plot.Fill/Pt. Color"=w166) -> ()  [unwired: 2 in, 2 out]
              }
            }
            n74 = Compound Arithmetic op=OR(w143, w142, w148) -> (w144:bool)
            n75 = case shown="True" w144 {
              tunnel: w145 -> [_ w173]
              tunnel: "Field Map" -> [_ w171]
              frame False {
              }
              frame True {
                # "load and display a field map"
                n76 = To Long Integer(number=w171) -> (32bit integer=w169:i32)
                n77 = Current VI's Path() -> (path=w176:path)
                n78 = Strip Path(path=w176) -> (stripped path=w175:path)  [unwired: 1 out]
                n79 = Strip Path(path=w175) -> (stripped path=w172:path)  [unwired: 1 out]
                n80 = List Folder(path=w172, pattern="*map*.png") -> (filenames=w170:string[])  [unwired: 2 in, 3 out]
                n81 = Index Array(array=w170, index=w169) -> (element=w168:string)
                n82 = property on="Field Map" class="Ring (strict)"("Strings []"=w170) -> ()  [unwired: 2 in, 2 out]
                n83 = Build Path(base path=w172, name or relative path=w168) -> (appended path=w174:path)
                n84 = call <vilib>:"Read PNG File.vi"("path to PNG file"=w174) -> ("error out"=w178:errorcluster, "image data"=w177:T18)  [unwired: 8 in, 1 out]
                n85 = case shown="No Error" w178 {
                  tunnel: w177 -> [w181 _]
                  tunnel: w173 -> [w196 _]
                  frame No Error {
                    w191 = T11 4 items=["Grayscale (U8)", "Grayscale (I16)", "Grayscale (SGL)", "Complex (CSG)", "RGB (U32)", "HSL (U32)", "RGB (U64)", "Grayscale (U16)"] ("Image Type")
                    w211 = T11 4 items=["Grayscale (U8)", "Grayscale (I16)", "Grayscale (SGL)", "Complex (CSG)", "RGB (U32)", "HSL (U32)", "RGB (U64)", "Grayscale (U16)"] ("Image Type")
                    n86 = call <vilib>:"Unflatten Pixmap.vi"("image data"=w181) -> ("24-bit pixmap"=w210:u32[][])  [unwired: 4 in, 6 out]
                    n87 = call <vilib>:"Unflatten Pixmap.vi"("image data"=w181) -> ("24-bit pixmap"=w190:u32[][])  [unwired: 4 in, 6 out]
                    n88 = property on="Robot Pose 1" class="XYGraph (strict)"() -> ("Width"=w214:u32, "Height"=w213:u32)  [unwired: 2 in, 2 out]
                    n89 = property on="Robot Pose 2" class="XYGraph (strict)"() -> ("Width"=w194:u32, "Height"=w193:u32)  [unwired: 2 in, 2 out]
                    n90 = call "IMAQ Create"("Image Name"="field1", "Image Type"=w211) -> ("New Image"=w209:T3)  [unwired: 3 in, 1 out]
                    n91 = call "IMAQ Create"("Image Name"="field2", "Image Type"=w191) -> ("New Image"=w189:T3)  [unwired: 3 in, 1 out]
                    n92 = Equal?(x=w196, y=WPI_DriverStationAllianceInfo."Red" ("x")) -> (x = y?=w198:bool)
                    n93 = call "IMAQ ArrayToColorImage"("Image Pixels (U32)"=w210, "Image"=w209) -> ("Image Out"=w208:T3)  [unwired: 3 in, 1 out]
                    n94 = call "IMAQ ArrayToColorImage"("Image Pixels (U32)"=w190, "Image"=w189) -> ("Image Out"=w188:T3)  [unwired: 3 in, 1 out]
                    n95 = To Long Integer(number=w214) -> (32bit integer=w204:i32)
                    n96 = To Long Integer(number=w213) -> (32bit integer=w205:i32)
                    n97 = To Long Integer(number=w194) -> (32bit integer=w184:i32)
                    n98 = To Long Integer(number=w193) -> (32bit integer=w185:i32)
                    n99 = call "IMAQ Resample"("X Resolution"=w204, "Y Resolution"=w205, "Image Src"=w208) -> ("Image Dst Out"=w203:T3)  [unwired: 7 in, 1 out]
                    n100 = call "IMAQ Resample"("X Resolution"=w184, "Y Resolution"=w185, "Image Src"=w188) -> ("Image Dst Out"=w183:T3)  [unwired: 7 in, 1 out]
                    n101 = Select(t=180.0, s=w198, f=0.0) -> (s? t:f=w201:dbl)
                    n102 = To Single Precision Float(number=w201) -> (single precision float=w179:sgl)
                    n103 = call "IMAQ Rotate"("Angle (degrees)"=w179, "Image Src"=w203) -> ("Image Dst Out"=w202:T3)  [unwired: 8 in, 1 out]
                    n104 = call "IMAQ Rotate"("Angle (degrees)"=w179, "Image Src"=w183) -> ("Image Dst Out"=w182:T3)  [unwired: 8 in, 1 out]
                    n105 = call "IMAQ ColorImageToArray"("Image"=w202) -> ("Image Pixels (U32)"=w207:u32[][])  [unwired: 3 in, 2 out]
                    n106 = call "IMAQ ColorImageToArray"("Image"=w182) -> ("Image Pixels (U32)"=w187:u32[][])  [unwired: 3 in, 2 out]
                    n107 = call <vilib>:"Flatten Pixmap.vi"("24-bit pixmap"=w207) -> ("image data"=w206:T18)  [unwired: 10 in]
                    n108 = call <vilib>:"Flatten Pixmap.vi"("24-bit pixmap"=w187) -> ("image data"=w186:T18)  [unwired: 10 in]
                    n109 = call <vilib>:"Draw Flattened Pixmap.vi"("image data"=w206) -> ("new picture"=w195:picture)  [unwired: 8 in]
                    n110 = call <vilib>:"Draw Flattened Pixmap.vi"("image data"=w186) -> ("new picture"=w180:picture)  [unwired: 8 in]
                    n111 = property on="Robot Pose 1" class="XYGraph (strict)"("PlotImages.Back"=w195) -> ()  [unwired: 2 in, 2 out]
                    n112 = property on="Robot Pose 2" class="XYGraph (strict)"("PlotImages.Back"=w180) -> ()  [unwired: 2 in, 2 out]
                  }
                  frame Error {
                  }
                }
              }
            }
            n113 = case shown="True" w149 {
              frame False {
              }
              frame True {
                # "export the current robot pose data"
                n114 = Get Date/Time In Seconds() -> (seconds since 1Jan1904=w228:timestamp)
                n115 = Format Date/Time String(time format string (%c)="%Y-%m-%d_%H-%M", seconds (now)=w228) -> (date/time string=w226:string)  [unwired: 1 in]
                n116 = Concatenate Strings("robot pose data " ("string"), w226) -> (w224:string)
                n117 = Current VI's Path() -> (path=w223:path)
                n118 = String To Path(string=w224) -> (path=w220:path)
                n119 = Strip Path(path=w223) -> (stripped path=w222:path)  [unwired: 1 out]
                n120 = Strip Path(path=w222) -> (stripped path=w221:path)  [unwired: 1 out]
                n121 = Build Path(base path=w221, name or relative path=w220) -> (appended path=w219:path)
                n122 = invoke on="Robot Pose 1" class="XYGraph (strict)" method="Export Image"("FileType"=enum32{"BMP", "EPS", "EMF", "PICT"}."BMP" ("File Type"), "Target"=enum32{"File", "Clipboard"}."File", "Path"=w219, "HideGrid"=TRUE ("Hide Grid"), "Overwrite"=TRUE ("Always Overwrite")) -> ()  [unwired: 3 in, 8 out]
              }
            }
            n123 = property on="Robot Pose 1" class="XYGraph (strict)"("XScale.Maximum"=w109, "YScale.Maximum"=w110) -> ()  [unwired: 2 in, 2 out]
            n124 = property on="Robot Pose 2" class="XYGraph (strict)"("XScale.Maximum"=w109, "YScale.Maximum"=w110) -> ()  [unwired: 2 in, 2 out]
            n125 = call-poly <vilib>:"NT Read Value.vi"("default value"=0.0 ("Default Value"), "name"="Robot_P" ("Name")) -> ("value"=→"Robot_P":dbl)  [unwired: 7 in, 2 out]
            n126 = call-poly <vilib>:"NT Read Value.vi"("default value"=0.0 ("Default Value"), "name"="Robot_H" ("Name")) -> ("value"=w160:dbl)  [unwired: 7 in, 2 out]
            n127 = call-poly <vilib>:"NT Read Value.vi"("default value"=-1.0 ("Default Value"), "name"="Robot_Y" ("Name")) -> ("value"=w106:dbl)  [unwired: 7 in, 2 out]
            "Robot_Y" <- w106
            n128 = call-poly <vilib>:"NT Read Value.vi"("default value"=-1.0 ("Default Value"), "name"="Robot_X" ("Name")) -> ("value"=w105:dbl)  [unwired: 7 in, 2 out]
            "Robot_X" <- w105
            n129 = call-poly <vilib>:"NT Read Value.vi"("default value"=dbl[] [0.0, 0.0, 0.0, 0.0] ("Default Value"), "name"="Targeting_Information" ("Name")) -> ("value"=w107:dbl[])  [unwired: 7 in, 2 out]
            n130 = call-poly <vilib>:"NT Read Value.vi"("default value"=30.0 ("Default Value"), "name"="Robot_Width_Bumpers" ("Name")) -> ("value"=w129:dbl)  [unwired: 7 in, 2 out]
            n131 = call-poly <vilib>:"NT Read Value.vi"("default value"=30.0 ("Default Value"), "name"="Robot_Length_Bumpers" ("Name")) -> ("value"=w130:dbl)  [unwired: 7 in, 2 out]
            n132 = Quotient & Remainder(x=w160, y=360.0) -> (x-y*floor(x/y)=→"Robot_H_GUI":dbl)  [unwired: 1 out]
            n133 = call-poly <vilib>:"NT Read Value.vi"("default value"=w87, "name"="Auto_Path_Xs" ("Name")) -> ("value"=w88:dbl[])  [unwired: 7 in, 2 out]
            n134 = call-poly <vilib>:"NT Read Value.vi"("default value"=w87, "name"="Auto_Path_Ys" ("Name")) -> ("value"=w90:dbl[])  [unwired: 7 in, 2 out]
            n135 = Bundle("value"=w90, "value"=w88) -> (w92:cluster{"value":dbl[], "value":dbl[]})  [unwired: 1 in]
            n136 = call "RenderRobotPose.vi"("Robot X (in)"=w105, "Robot Width (in)"=w129, "Robot Length (in)"=w130, "Buffer Time (min)"=0.5, "Robot Y (in)"=w106, "Targeting Information"=w107, "Robot Heading (deg)"=w160, "Planned Path"=w92, "Robot Enabled"=TRUE, "Reset"="Clear_Robot_Pose_Display") -> ("Robot Pose"=→"Robot Pose 2" →"Robot Pose 1":cluster{dbl[], dbl[]}[])  [unwired: 5 in]
            n137 = local read "No_Secondary_Camera"() -> (w123:bool)
            n138 = property on="Robot Pose 2" class="XYGraph (strict)"("Visible"=w123) -> ()  [unwired: 2 in, 2 out]
            n139 = call-poly <vilib>:"NT Read Value.vi"("default value"=FALSE, "name"="Pointed_at_Target" ("Name")) -> ("value"=→"Pointed_at_Target":bool)  [unwired: 7 in, 2 out]
            n140 = call-poly <vilib>:"NT Read Value.vi"("name"="LL_Valid" ("Name")) -> ("value"=→"LL_Valid":bool)  [unwired: 8 in, 2 out]
            n141 = call-poly <vilib>:"NT Read Value.vi"("name"="Vision_Fault" ("Name")) -> ("value"=→"Vision_Fault_GUI":bool)  [unwired: 8 in, 2 out]
            n142 = call-poly <vilib>:"NT Read Value.vi"("default value"=0.0, "name"="Distance_to_Target" ("Name")) -> ("value"=→"Distance_to_Target":dbl)  [unwired: 7 in, 2 out]
            n143 = call-poly <vilib>:"NT Read Value.vi"("default value"=0.0, "name"="Heading_to_Target" ("Name")) -> ("value"=→"Heading_to_Target":dbl)  [unwired: 7 in, 2 out]
          }
          frame #2 {
            # "driver control configuration"
            # "robot configuration"
            # "robot and driver control configuration"
            n144 = local read "Dashboard Tab"() -> (w229:T1)
            n145 = case shown="\"Setup/Auto\"" w229 {
              frame "Checklist", Default {
              }
              frame "Setup/Auto" {
                n146 = call-poly <vilib>:"NT Read Value.vi"("default value"="No robot profile..." ("Default Value"), "name"="Robot_Profile" ("Name")) -> ("value"=→"Robot_Profile_GUI":string)  [unwired: 7 in, 2 out]
              }
            }
            n147 = Build Array("N/A") -> (w240:string[])
            n148 = And(x="Calibrate_Joysticks_GUI", y="Arm_Calibrate_Joysticks") -> (x .and. y?=w230:bool)
            n149 = To Double Precision Float(number="Select Driver Profile") -> (double precision float=w233:dbl)
            n150 = call-poly <vilib>:"NT Read Value.vi"("default value"=w240, "name"="Legal_Drivers" ("Name")) -> ("value"=w239:string[])  [unwired: 7 in, 2 out]
            "Legal_Drivers_GUI" <- w239
            n151 = Not(x="Arm_Calibrate_Joysticks") -> (.not. x?=w242:bool)
            n152 = call "ReducedBWSendToNT.vim"("Value In"=w233, "NT Name"="Selected_Driver" ("Name")) -> ()  [unwired: 1 out]
            n153 = property on="Select Driver Profile" class="Ring (strict)"("Strings []"=w239) -> ()  [unwired: 2 in, 2 out]
            n154 = call "ReducedBWSendToNT.vim"("Value In"=w230, "NT Name"="Calibrate_Joysticks" ("Name")) -> ()  [unwired: 1 out]
            n155 = Select(t=cluster{u32, u32}[] [{11776947, 16448250}, {16448250, 16448250}] ("Colors [4]"), s=w242, f=cluster{u32, u32}[] [{6618880, 16448250}, {16448250, 16448250}] ("Colors [4]")) -> (s? t:f=w243:cluster{u32, u32}[])
            n156 = property on="Calibrate_Joysticks_GUI" class="Bool"("Colors [4]"=w243) -> ()  [unwired: 2 in, 2 out]
          }
          frame #3 {
            # "configure auto play"
            # "set robot pose"
            # "autonomous configuration"
            n157 = call "ReducedBWSendToNT.vim"("Value In"="Manual_Start_X", "NT Name"="Manual_Start_X" ("Name")) -> ()  [unwired: 1 out]
            n158 = call "ReducedBWSendToNT.vim"("Value In"="Manual_Start_Y", "NT Name"="Manual_Start_Y" ("Name")) -> ()  [unwired: 1 out]
            n159 = call "ReducedBWSendToNT.vim"("Value In"="Manual_Start_H", "NT Name"="Manual_Start_H" ("Name")) -> ()  [unwired: 1 out]
            n160 = call "ReducedBWSendToNT.vim"("Value In"="Disable_Fusion_While_Autonomous", "NT Name"="Disable_Fusion_While_Autonomous" ("Name")) -> ()  [unwired: 1 out]
            n161 = call "ReducedBWSendToNT.vim"("Value In"="Disable_Fusion_While_Disabled", "NT Name"="Disable_Fusion_While_Disabled" ("Name")) -> ()  [unwired: 1 out]
            n162 = call "ReducedBWSendToNT.vim"("Value In"="Push_Robot_Start_GUI", "NT Name"="Push_Robot_Start" ("Name")) -> ()  [unwired: 1 out]
            n163 = local read "Dashboard Tab"() -> (w250:T1)
            n164 = To Double Precision Float(number="Select Autonomous Play") -> (double precision float=w253:dbl)
            n165 = call "ReducedBWSendToNT.vim"("Value In"="Auto_Test_Mode_GUI", "NT Name"="Auto_Test_Mode" ("Name")) -> ()  [unwired: 1 out]
            n166 = call "ReducedBWSendToNT.vim"("Value In"="Auto_Delay_GUI", "NT Name"="Auto_Delay" ("Name")) -> ()  [unwired: 1 out]
            n167 = call "ReducedBWSendToNT.vim"("Value In"="Force_Human_Control_GUI", "NT Name"="Force_Human_Control" ("Name")) -> ()  [unwired: 1 out]
            n168 = call "ReducedBWSendToNT.vim"("Value In"=w253, "NT Name"="Selected_Auto_Play" ("Name")) -> ()  [unwired: 1 out]
            n169 = call "ReducedBWSendToNT.vim"("Value In"="Refresh_Auto_Play_List_GUI", "NT Name"="Refresh_Auto_Play_List" ("Name")) -> ()  [unwired: 1 out]
            n170 = case shown="\"Setup/Auto\"" w250 {
              tunnel: "Select Autonomous Play" -> [_ w273]
              tunnel: "Refresh_Auto_Play_List_GUI" -> [_ w272]
              frame "Checklist", Default {
              }
              frame "Setup/Auto" {
                w290 = "N/A" ("Default Value")
                n171 = call-poly <vilib>:"NT Read Value.vi"("default value"=0.0, "name"="Suggested_Start_H" ("Name")) -> ("value"=w289:dbl)  [unwired: 7 in, 2 out]
                n172 = call-poly <vilib>:"NT Read Value.vi"("default value"=0.0, "name"="Suggested_Start_X" ("Name")) -> ("value"=w287:dbl)  [unwired: 7 in, 2 out]
                n173 = call-poly <vilib>:"NT Read Value.vi"("default value"=0.0, "name"="Suggested_Start_Y" ("Name")) -> ("value"=w288:dbl)  [unwired: 7 in, 2 out]
                n174 = Build Array("N/A") -> (w293:string[])
                n175 = call "Is Value Changed.vim"("value"=w273) -> ("changed or first call?"=w274:bool)
                n176 = call "Is Value Changed.vim"("value"=w289) -> ("changed or first call?"=w280:bool)
                n177 = call "Is Value Changed.vim"("value"=w287) -> ("changed or first call?"=w276:bool)
                n178 = call "Is Value Changed.vim"("value"=w288) -> ("changed or first call?"=w278:bool)
                n179 = call-poly <vilib>:"NT Read Value.vi"("default value"=w290, "name"="Auto_Playbook" ("Name")) -> ("value"=→"Auto_Playbook_GUI":string)  [unwired: 7 in, 2 out]
                n180 = call-poly <vilib>:"NT Read Value.vi"("default value"=w290, "name"="Auto_Path_Suffix" ("Name")) -> ("value"=→"Auto_Suffix_GUI":string)  [unwired: 7 in, 2 out]
                n181 = call-poly <vilib>:"NT Read Value.vi"("default value"=w293, "name"="Legal_Auto_Plays" ("Name")) -> ("value"=w294:string[])  [unwired: 7 in, 2 out]
                n182 = Compound Arithmetic op=OR(w274, w272, w276) -> (w275:bool)
                n183 = Compound Arithmetic op=OR(w274, w272, w278) -> (w277:bool)
                n184 = Compound Arithmetic op=OR(w274, w272, w280) -> (w279:bool)
                n185 = property on="Select Autonomous Play" class="Ring (strict)"("Strings []"=w294) -> ()  [unwired: 2 in, 2 out]
                n186 = case shown="True" w279 {
                  tunnel: w289 -> [_ w299]
                  frame False {
                  }
                  frame True {
                    n187 = property on="Manual_Start_H" class="DigNum (strict)"("Value"=w299) -> ()  [unwired: 2 in, 2 out]
                  }
                }
                n188 = case shown="True" w277 {
                  tunnel: w288 -> [_ w300]
                  frame False {
                  }
                  frame True {
                    n189 = property on="Manual_Start_Y" class="DigNum (strict)"("Value"=w300) -> ()  [unwired: 2 in, 2 out]
                  }
                }
                n190 = case shown="True" w275 {
                  tunnel: w287 -> [_ w301]
                  frame False {
                  }
                  frame True {
                    n191 = property on="Manual_Start_X" class="DigNum (strict)"("Value"=w301) -> ()  [unwired: 2 in, 2 out]
                  }
                }
              }
            }
          }
          frame #4 {
            w317 = bool[] [FALSE, FALSE, FALSE, FALSE, FALSE, FALSE] ("default value")
            w316 = bool[] [FALSE, FALSE, FALSE, FALSE, FALSE, FALSE] ("Default Value")
            w318 = cluster{u32, u32}[] [{9567230, 16448250}, {16448250, 16448250}] ("Un-selected Color")
            # "master state controller"
            # "state indicators"
            n192 = global read "GlobalDashboard.vi" "Code_is_Running"() -> (w315:bool)
            n193 = call-poly <vilib>:"NT Read Value.vi"("default value"=w317, "name"="Confirmed_States" ("Name")) -> ("value"=w312:bool[])  [unwired: 7 in, 2 out]
            n194 = call-poly <vilib>:"NT Read Value.vi"("default value"=w316, "name"="Disallowed_States" ("Name")) -> ("value"=w314:bool[])  [unwired: 7 in, 2 out]
            n195 = Select(t=w314, s=w315, f=w316) -> (s? t:f=w313:bool[])
            n196 = Select(t=w312, s=w315, f=w317) -> (s? t:f=w311:bool[])
            n197 = Index Array(array=w313, index #1=0 ("index")) -> (element #1=w323:bool, element #2=w322:bool, element #3=w320:bool, element #4=w319:bool)  [unwired: 3 in]
            n198 = Index Array(array=w311, index #1=0 ("index")) -> (element #1=w329:bool, element #2=w325:bool, element #3=w310:bool, element #4=w309:bool, element #5=→"State_Shelf":bool)  [unwired: 4 in]
            "State_Score" <- w310
            "State_Hopper" <- w309
            n199 = call "ButtonColorChooser.vi"("Un-selected Color"=w318, "Disallowed"=w323, "Confirmed"=w329) -> ("Final Color"=w330:cluster{u32, u32}[])  [unwired: 8 in]
            n200 = call "ButtonColorChooser.vi"("Un-selected Color"=w318, "Disallowed"=w322, "Confirmed"=w325) -> ("Final Color"=w305:cluster{u32, u32}[])  [unwired: 8 in]
            n201 = call "ButtonColorChooser.vi"("Un-selected Color"=w318, "Disallowed"=w320, "Confirmed"=w310) -> ("Final Color"=w304:cluster{u32, u32}[])  [unwired: 8 in]
            n202 = call "ButtonColorChooser.vi"("Un-selected Color"=w318, "Disallowed"=w319, "Confirmed"=w309) -> ("Final Color"=w303:cluster{u32, u32}[])  [unwired: 8 in]
            n203 = property on="Master_State_SPEAKER_Indicator" class="Bool (strict)"("Colors [4]"=w330) -> ()  [unwired: 2 in, 2 out]
            n204 = property on="Master_State_AMP_Indicator" class="Bool (strict)"("Colors [4]"=w305) -> ()  [unwired: 2 in, 2 out]
            n205 = property on="Master_State_CLIMB_Indicator" class="Bool (strict)"("Colors [4]"=w304) -> ()  [unwired: 2 in, 2 out]
            n206 = property on="Master_State_TRAP_Indicator" class="Bool (strict)"("Colors [4]"=w303) -> ()  [unwired: 2 in, 2 out]
            "Master_State_SPEAKER_Indicator" <- FALSE ("Master_State_0_Indicator")
            "Master_State_AMP_Indicator" <- FALSE ("Master_State_0_Indicator")
            "Master_State_CLIMB_Indicator" <- FALSE ("Master_State_0_Indicator")
            "Master_State_TRAP_Indicator" <- FALSE ("Master_State_0_Indicator")
          }
          frame #5 {
            # "actuator test interlocks"
            # "emergency overrides"
            # "emergency overrides and interlocks"
            n207 = global read "GlobalDashboard.vi" "Code_is_Running"() -> (w334:bool)
            n208 = call-poly <vilib>:"NT Read Value.vi"("default value"=FALSE, "name"="Robot_in_Safety_Override" ("Name")) -> ("value"=w336:bool)  [unwired: 7 in, 2 out]
            n209 = call "EdgeTrigger.vi"("Input Signal"=w336) -> ("All Edge Trigger"=w337:bool)  [unwired: 2 out]
            n210 = call "EdgeTrigger.vi"("Input Signal"=w334) -> ("Falling Edge Trigger"=w333:bool)  [unwired: 2 out]
            n211 = call "ReducedBWSendToNT.vim"("Value In"="Clear_Errors_GUI", "NT Name"="Clear_Errors" ("Name")) -> ()  [unwired: 1 out]
            n212 = call "ReducedBWSendToNT.vim"("Value In"="Super_Test_Mode_GUI", "NT Name"="Super_Test_Mode" ("Name")) -> ()  [unwired: 1 out]
            n213 = call "ReducedBWSendToNT.vim"("Value In"="Auto_Targeting_Override", "NT Name"="Auto_Targeting_Override" ("Name")) -> ()  [unwired: 1 out]
            n214 = call "ReducedBWSendToNT.vim"("Value In"="Camera_Override_GUI", "NT Name"="Camera_Override" ("Name")) -> ()  [unwired: 1 out]
            n215 = call "ReducedBWSendToNT.vim"("Value In"="Field_Oriented_Override_GUI", "NT Name"="Field_Oriented_Override" ("Name")) -> ()  [unwired: 1 out]
            n216 = case shown="True" w337 {
              tunnel: w336 -> [_ w362]
              frame False {
              }
              frame True {
                n217 = property on="Master_Safety_Override_1" class="Bool (strict)"("Value"=w362) -> ()  [unwired: 2 in, 2 out]
              }
            }
            n218 = case shown="True" w333 {
              frame False {
              }
              frame True {
                n219 = property on="Master_Safety_Override_1" class="Bool (strict)"("Value"=FALSE ("Master_Safety_Override_1")) -> ()  [unwired: 2 in, 2 out]
              }
            }
            n220 = call "ReducedBWSendToNT.vim"("Value In"="Master_Safety_Override_1", "NT Name"="Master_Safety_Override" ("Name")) -> ()  [unwired: 1 out]
            n221 = property on="Actuator Testing" class="Ring (strict)"() -> ("RingText.Text"=w346:string)  [unwired: 2 in, 2 out]
            n222 = Build Array("No_Test") -> (w360:string[])
            n223 = call "ReducedBWSendToNT.vim"("Value In"="Free_Tuning_Variable_GUI", "NT Name"="Free_Tuning_Variable" ("Name")) -> ()  [unwired: 1 out]
            n224 = call-poly <vilib>:"NT Read Value.vi"("default value"=w360, "name"="Legal_Actuator_Names" ("Name")) -> ("value"=w359:string[])  [unwired: 7 in, 2 out]
            n225 = call "ReducedBWSendToNT.vim"("Value In"=w346, "NT Name"="Test_Actuator_Name" ("Name")) -> ()  [unwired: 1 out]
            n226 = call "ReducedBWSendToNT.vim"("Value In"="Test_Actuator_Value_GUI", "NT Name"="Test_Actuator_Value" ("Name")) -> ()  [unwired: 1 out]
            n227 = call "ReducedBWSendToNT.vim"("Value In"="Test_Actuator_Period_GUI", "NT Name"="Test_Actuator_Period" ("Name")) -> ()  [unwired: 1 out]
            n228 = property on="Actuator Testing" class="Ring (strict)"("Strings []"=w359) -> ()  [unwired: 2 in, 2 out]
          }
          frame #6 {
            # "drivebase subsytem"
            n229 = call "SwerveModuleReadData.vi"("NT Name (Errors)"="Swerve_1_Errors", "NT Name (Details)"="Swerve_1_Details" ("NT Name (Tune)")) -> ("Shifter State"=→"Swerve_1_Shifter_State":string, "Drive Velocity"=→"Swerve_1_Drive_Velocity":dbl, "Drive Temperature"=→"Swerve_1_Drive_Temperature":dbl, "Azimuth Position"=→"Swerve_1_Azimuth_Position":dbl, "Shifter Failure"=w429:T19, "Drive Overheating"=w431:T19, "Drive Fault"=w376:T19, "Azimuth Fault"=w430:T19)  [unwired: 2 in]
            n230 = call "SwerveModuleReadData.vi"("NT Name (Errors)"="Swerve_0_Errors", "NT Name (Details)"="Swerve_0_Details" ("NT Name (Tune)")) -> ("Shifter State"=→"Swerve_0_Shifter_State":string, "Drive Velocity"=→"Swerve_0_Drive_Velocity":dbl, "Drive Temperature"=→"Swerve_0_Drive_Temperature":dbl, "Azimuth Position"=→"Swerve_0_Azimuth_Position":dbl, "Shifter Failure"=w437:T19, "Drive Overheating"=w445:T19, "Drive Fault"=w378:T19, "Azimuth Fault"=w441:T19)  [unwired: 2 in]
            n231 = call-poly <vilib>:"NT Read Value.vi"("name"="IMU_Failure" ("Name")) -> ("value"=→"IMU_Failure_GUI":bool)  [unwired: 8 in, 2 out]
            n232 = call-poly <vilib>:"NT Read Value.vi"("name"="Field_Oriented" ("Name")) -> ("value"=→"Field_Oriented_GUI":bool)  [unwired: 8 in, 2 out]
            n233 = call "SwerveModuleReadData.vi"("NT Name (Errors)"="Swerve_2_Errors", "NT Name (Details)"="Swerve_2_Details" ("NT Name (Tune)")) -> ("Shifter State"=→"Swerve_2_Shifter_State":string, "Drive Velocity"=→"Swerve_2_Drive_Velocity":dbl, "Drive Temperature"=→"Swerve_2_Drive_Temperature":dbl, "Azimuth Position"=→"Swerve_2_Azimuth_Position":dbl, "Shifter Failure"=w424:T19, "Drive Overheating"=w426:T19, "Drive Fault"=w374:T19, "Azimuth Fault"=w425:T19)  [unwired: 2 in]
            n234 = call "SwerveModuleReadData.vi"("NT Name (Errors)"="Swerve_3_Errors", "NT Name (Details)"="Swerve_3_Details" ("NT Name (Tune)")) -> ("Shifter State"=→"Swerve_3_Shifter_State":string, "Drive Velocity"=→"Swerve_3_Drive_Velocity":dbl, "Drive Temperature"=→"Swerve_3_Drive_Temperature":dbl, "Azimuth Position"=→"Swerve_3_Azimuth_Position":dbl, "Shifter Failure"=w419:T19, "Drive Overheating"=w421:T19, "Drive Fault"=w372:T19, "Azimuth Fault"=w420:T19)  [unwired: 2 in]
            n235 = Unbundle(w431) -> ("Boolean"=w417:bool, "Numeric Text.Text Colors:Text Color"=w414:u32)
            n236 = Unbundle(w430) -> ("Boolean"=w418:bool, "Numeric Text.Text Colors:Text Color"=w415:u32)
            n237 = Unbundle(w445) -> ("Boolean"=w443:bool, "Numeric Text.Text Colors:Text Color"=w444:u32)
            n238 = Unbundle(w441) -> ("Boolean"=w440:bool, "Numeric Text.Text Colors:Text Color"=w438:u32)
            n239 = Unbundle(w429) -> ("Boolean"=w416:bool, "Numeric Text.Text Colors:Text Color"=w409:u32)
            n240 = Unbundle(w426) -> ("Boolean"=w407:bool, "Numeric Text.Text Colors:Text Color"=w405:u32)
            n241 = Unbundle(w437) -> ("Boolean"=w435:bool, "Numeric Text.Text Colors:Text Color"=w436:u32)
            n242 = Unbundle(w378) -> ("Boolean"=w370:bool, "Numeric Text.Text Colors:Text Color"=w379:u32)
            n243 = Unbundle(w425) -> ("Boolean"=w408:bool, "Numeric Text.Text Colors:Text Color"=w406:u32)
            n244 = Unbundle(w421) -> ("Boolean"=w396:bool, "Numeric Text.Text Colors:Text Color"=w395:u32)
            n245 = Unbundle(w420) -> ("Boolean"=w397:bool, "Numeric Text.Text Colors:Text Color"=w398:u32)
            n246 = Unbundle(w376) -> ("Boolean"=w369:bool, "Numeric Text.Text Colors:Text Color"=w377:u32)
            n247 = Unbundle(w424) -> ("Boolean"=w400:bool, "Numeric Text.Text Colors:Text Color"=w399:u32)
            n248 = Unbundle(w374) -> ("Boolean"=w368:bool, "Numeric Text.Text Colors:Text Color"=w375:u32)
            n249 = Unbundle(w419) -> ("Boolean"=w389:bool, "Numeric Text.Text Colors:Text Color"=w390:u32)
            n250 = Unbundle(w372) -> ("Boolean"=w367:bool, "Numeric Text.Text Colors:Text Color"=w373:u32)
            n251 = property on="Swerve_0_Shifter_State" class="Str"("Text.BG Color"=w436) -> ()  [unwired: 2 in, 2 out]
            n252 = property on="Swerve_1_Shifter_State" class="Str"("Text.BG Color"=w409) -> ()  [unwired: 2 in, 2 out]
            n253 = property on="Swerve_2_Shifter_State" class="Str"("Text.BG Color"=w399) -> ()  [unwired: 2 in, 2 out]
            n254 = property on="Swerve_3_Shifter_State" class="Str"("Text.BG Color"=w390) -> ()  [unwired: 2 in, 2 out]
            n255 = property on="Swerve_3_Drive_Velocity" class="DigNum (strict)"("NumText.BG Color"=w373) -> ()  [unwired: 2 in, 2 out]
            n256 = property on="Swerve_0_Azimuth_Position" class="DigNum (strict)"("NumText.BG Color"=w438) -> ()  [unwired: 2 in, 2 out]
            n257 = property on="Swerve_0_Drive_Temperature" class="DigNum (strict)"("NumText.BG Color"=w444) -> ()  [unwired: 2 in, 2 out]
            n258 = property on="Swerve_1_Azimuth_Position" class="DigNum (strict)"("NumText.BG Color"=w415) -> ()  [unwired: 2 in, 2 out]
            n259 = property on="Swerve_1_Drive_Temperature" class="DigNum (strict)"("NumText.BG Color"=w414) -> ()  [unwired: 2 in, 2 out]
            n260 = property on="Swerve_2_Azimuth_Position" class="DigNum (strict)"("NumText.BG Color"=w406) -> ()  [unwired: 2 in, 2 out]
            n261 = property on="Swerve_2_Drive_Temperature" class="DigNum (strict)"("NumText.BG Color"=w405) -> ()  [unwired: 2 in, 2 out]
            n262 = property on="Swerve_3_Azimuth_Position" class="DigNum (strict)"("NumText.BG Color"=w398) -> ()  [unwired: 2 in, 2 out]
            n263 = property on="Swerve_3_Drive_Temperature" class="DigNum (strict)"("NumText.BG Color"=w395) -> ()  [unwired: 2 in, 2 out]
            n264 = property on="Swerve_0_Drive_Velocity" class="DigNum (strict)"("NumText.BG Color"=w379) -> ()  [unwired: 2 in, 2 out]
            n265 = property on="Swerve_2_Drive_Velocity" class="DigNum (strict)"("NumText.BG Color"=w375) -> ()  [unwired: 2 in, 2 out]
            n266 = property on="Swerve_1_Drive_Velocity" class="DigNum (strict)"("NumText.BG Color"=w377) -> ()  [unwired: 2 in, 2 out]
            n267 = call-poly <vilib>:"NT Read Value.vi"("name"="Using_Auto_Targeting" ("Name")) -> ("value"=→"Using_Auto_Targeting":bool)  [unwired: 8 in, 2 out]
            n268 = Build Array(w435, w416, w400, w389) -> (→"Swerve_Shifter_Failure_Array":bool[])
            n269 = Build Array(w440, w418, w408, w397) -> (→"Swerve_Azimuth_Fault_Array":bool[])
            n270 = Build Array(w443, w417, w407, w396) -> (→"Swerve_Overheating_Array":bool[])
            n271 = Build Array(w370, w369, w368, w367) -> (→"Swerve_Drive_Fault_Array":bool[])
            n272 = local read "Dashboard Tab"() -> (w380:T1)
            n273 = case shown="\"Tune\"" w380 {
              frame "Checklist", Default {
              }
              frame "Tune" {
                n274 = call-poly <vilib>:"NT Read Value.vi"("default value"=dbl[] [0.0, 0.0, 0.0, 0.0, 0.0, 0.0] ("Default Value"), "name"="Current_Driver_Profile_Setpoints" ("Name")) -> ("value"=w470:dbl[])  [unwired: 7 in, 2 out]
                n275 = Array To Cluster(array=w470) -> (cluster=w466:T20)
                "Current_Driver_Profile_Setpoints_GUI" <- w466
                n276 = feedback #3(dbl[] [0.0, 0.0, 0.0, 0.0, 0.0, 0.0] ("Default Value")) -> (w469:dbl[])
                n277 = feedback-in #3(w470) -> ()
                n278 = Not Equal?(x=w470, y=w469) -> (x != y?=w468:bool[])
                n279 = Or Array Elements(Boolean array=w468) -> (logical OR=w467:bool)
                n280 = case shown="True" w467 {
                  tunnel: w466 -> [_ w474]
                  frame False {
                  }
                  frame True {
                    n281 = property on="New_Driver_Profile_Setpoints_GUI" class="Clust (strict)"("Value"=w474) -> ()  [unwired: 2 in, 2 out]
                  }
                }
              }
            }
            n282 = local read "Select Driver Profile"() -> (w454:u16)
            n283 = local read "Legal_Drivers_GUI"() -> (w455:string[])
            n284 = Cluster To Array(cluster="New_Driver_Profile_Setpoints_GUI") -> (array=w384:dbl[])
            n285 = And(x="Calibrate_Wheels_GUI", y="Arm_Calibrate_Wheels_GUI") -> (x .and. y?=w387:bool)
            n286 = Not(x="Arm_Calibrate_Wheels_GUI") -> (.not. x?=w461:bool)
            n287 = To Long Integer(number=w454) -> (32bit integer=w452:i32)
            n288 = call "ReducedBWSendToNT.vim"("Value In"="Home_Wheels_GUI", "NT Name"="Home_Wheels" ("Name")) -> ()  [unwired: 1 out]
            n289 = Index Array(array=w455, index=w452) -> (element=→"Current_Driver_Profile_GUI":string)
            n290 = call "ReducedBWSendToNT.vim"("Value In"="Apply_Driver_Profile_Setpoints_GUI", "NT Name"="Apply_Driver_Profile_Setpoints" ("Name")) -> ()  [unwired: 1 out]
            n291 = call "ReducedBWSendToNT.vim"("Value In"=w384, "NT Name"="New_Driver_Profile_Setpoints" ("Name")) -> ()  [unwired: 1 out]
            n292 = call "ReducedBWSendToNT.vim"("Value In"=w387, "NT Name"="Calibrate_Wheels" ("Name")) -> ()  [unwired: 1 out]
            n293 = call "ReducedBWSendToNT.vim"("Value In"="Arm_Calibrate_Wheels_GUI", "NT Name"="Unlock_Azimuth") -> ()  [unwired: 1 out]
            n294 = Select(t=cluster{u32, u32}[] [{11776947, 16448250}, {16448250, 16448250}] ("Colors [4]"), s=w461, f=cluster{u32, u32}[] [{6618880, 16448250}, {16448250, 16448250}] ("Colors [4]")) -> (s? t:f=w460:cluster{u32, u32}[])
            n295 = property on="Calibrate_Wheels_GUI" class="Bool"("Colors [4]"=w460) -> ()  [unwired: 2 in, 2 out]
          }
          frame #7 {
            # "arm and gripper subsystem"
          }
          frame #8 {
            # "intake subsystem"
          }
          frame #9 {
            # "combine errors for in-match reporting"
            # "manage targeting reticules"
            # "manage audible warnings"
            # "error management and driver assistance"
            n296 = local read "Swerve_Azimuth_Fault_Array"() -> (w501:bool[])
            n297 = local read "Swerve_Shifter_Failure_Array"() -> (w504:bool[])
            n298 = local read "Swerve_Overheating_Array"() -> (w502:bool[])
            n299 = local read "Swerve_Drive_Fault_Array"() -> (w480:bool[])
            n300 = Or Array Elements(Boolean array=w501) -> (logical OR=→"Swerve_Azimuth_Fault":bool)
            n301 = Or Array Elements(Boolean array=w502) -> (logical OR=→"Swerve_Overheating":bool)
            n302 = Or Array Elements(Boolean array=w504) -> (logical OR=→"Swerve_Shifter_Failure":bool)
            n303 = Or Array Elements(Boolean array=w480) -> (logical OR=→"Swerve_Drive_Fault":bool)
            n304 = Build Array("Driver_Help", "Manipulator_Help") -> (w509:bool[])
            n305 = Or Array Elements(Boolean array=w509) -> (logical OR=w500:bool)
            n306 = Not(x=w500) -> (.not. x?=w517:bool)
            n307 = Build Array (concatenate)(w517, w509) -> (w516:bool[])
            n308 = property on="Help Graphic" class="ImageControl"("Visible"=w500) -> ()  [unwired: 2 in, 2 out]
            n309 = call "StateSelection.vi"("Disallowed States"=bool[] [FALSE, FALSE, FALSE, FALSE], "State Triggers"=w516, "State Names"=string[] ["No Help", "Driver Help", "Manipulator Help"]) -> ("Selected State"=w521:string)
            n310 = case shown="\"Driver Help\"" w521 {
              tunnel: [_ w542 w544] -> w503
              tunnel: w500 -> [_ _ _]
              frame "No Help", Default {
              }
              frame "Driver Help" {
                n311 = call "RenderJoystickDiagram.vi"("Joystick Graphic Filename"="driver joystick diagram.png") -> ("Image Out"=w542:T3)  [unwired: 10 in]
              }
              frame "Manipulator Help" {
                n312 = call "RenderJoystickDiagram.vi"("Joystick Graphic Filename"="manipulator joystick diagram.png") -> ("Image Out"=w544:T3)  [unwired: 10 in]
              }
            }
            "Help Graphic" <- w503
            n313 = Or Array Elements(Boolean array=w509) -> (logical OR=w511:bool)
            n314 = Not(x=w511) -> (.not. x?=w510:bool)
            n315 = Or(x=w510, y=w509) -> (x .or. y?=w508:bool[])
            n316 = Index Array(array=w508) -> (element #1=w482:bool, element #2=w481:bool)  [unwired: 2 in]
            n317 = Select(t=T13."Enabled" ("Disabled"), s=w481, f=T13."Disabled and Grayed Out" ("Disabled")) -> (s? t:f=w512:T13)
            n318 = Select(t=T13."Enabled" ("Disabled"), s=w482, f=T13."Disabled and Grayed Out" ("Disabled")) -> (s? t:f=w541:T13)
            n319 = property on="Driver_Help" class="Bool (strict)"("DisabledEnum"=w541) -> ()  [unwired: 2 in, 2 out]
            n320 = property on="Manipulator_Help" class="Bool (strict)"("DisabledEnum"=w512) -> ()  [unwired: 2 in, 2 out]
            n321 = First Call?() -> (First Call?: T/F=w489:bool)
            n322 = call-poly <vilib>:"NT Read Value.vi"("default value"=FALSE ("Default Value"), "name"="Master_Alarm" ("Name")) -> ("value"=w485:bool)  [unwired: 7 in, 2 out]
            n323 = call "Timer.vi"("Reset Timer"=w489) -> ("Time (ms)"=w488:u32)
            n324 = Greater?(x=w488, y=u32 2500) -> (0:w486:bool)
            n325 = local read "Arm_Calibrate_Wheels_GUI"() -> (w491:bool)
            n326 = call-poly <vilib>:"NT Read Value.vi"("default value"=0.0 ("Default Value"), "name"="Number_of_Master_Alarms" ("Name")) -> ("value"=w495:dbl)  [unwired: 7 in, 2 out]
            n327 = And(x=w486, y=w485) -> (x .and. y?=w484:bool)
            n328 = call "EdgeTrigger.vi"("Input Signal"="Mute_Audible_Warnings") -> ("Rising Edge Trigger"=w529:bool)  [unwired: 2 out]
            n329 = local read "Arm_Calibrate_Joysticks"() -> (w492:bool)
            n330 = To Long Integer(number=w495) -> (32bit integer=w494:i32)
            n331 = call "BlinkLight.vi"() -> ("Blinked"=w534:bool)  [unwired: 1 in]
            n332 = Number To Decimal String(number=w494) -> (decimal integer string=w535:string)  [unwired: 1 in]
            n333 = feedback #4(TRUE ("t")) -> (w527:bool)
            n334 = Not(x=w527) -> (.not. x?=w526:bool)
            n335 = Select(t=w526, s=w529, f=w527) -> (s? t:f=w483:bool)
            "Audible_Warnings_Enabled_GUI" <- w483
            n336 = feedback-in #4(w483) -> ()
            n337 = Select(t=w534, s=w484, f=FALSE) -> (s? t:f=w538:bool)
            "Master_Caution_GUI_1" <- w538
            "Master_Caution_GUI_0" <- w538
            "Master_Caution_GUI_2" <- w538
            n338 = Concatenate Strings("MASTER ALARM (" ("string"), w535, ")" ("string")) -> (w536:string)
            n339 = Select(t=w536, s=w538, f="") -> (s? t:f=w537:string)
            n340 = Compound Arithmetic op=OR(w492, w491) -> (w490:bool)
            n341 = local read "State_Hopper"() -> (→"WA_Ret_Left" →"WA_Ret_Right":bool)
            n342 = Select(t=cluster{u32, u32}[] [{6618880, 16448250}, {16448250, 16448250}] ("Colors [4]"), s=w483, f=cluster{u32, u32}[] [{16755474, 16448250}, {16448250, 16448250}] ("Colors [4]")) -> (s? t:f=w525:cluster{u32, u32}[])
            n343 = local read "State_Score"() -> (w477:bool)
            n344 = local read "State_Shelf"() -> (w476:bool)
            n345 = call "ReducedBWSendToNT.vim"("Value In"=w490, "NT Name"="Some_Switch_Armed" ("Name")) -> ()  [unwired: 1 out]
            n346 = property on="Master_Caution_GUI_0" class="Bool (strict)"("BoolText.Text"=w537) -> ()  [unwired: 2 in, 2 out]
            n347 = property on="Master_Caution_GUI_1" class="Bool (strict)"("BoolText.Text"=w537) -> ()  [unwired: 2 in, 2 out]
            n348 = property on="Master_Caution_GUI_2" class="Bool (strict)"("BoolText.Text"=w537) -> ()  [unwired: 2 in, 2 out]
            n349 = property on="Mute_Audible_Warnings" class="Bool"("Colors [4]"=w525) -> ()  [unwired: 2 in, 2 out]
            n350 = Or(x=w477, y=w476) -> (x .or. y?=→"LL_Ret_Left" →"LL_Ret_Right":bool)
          }
          frame #10 {
            # "flush NT tables"
            n351 = call <vilib>:"NT Flush Data Updates.vi"() -> ()  [unwired: 11 in, 1 out]
          }
        }
      }
    }
  }
  n352 = while {
    stop <- FALSE stop-if-true
    # "Set window properties"
    n353 = Not(x="Dock_Dashboard") -> (.not. x?=w547:bool)
    n354 = First Call?() -> (First Call?: T/F=w551:bool)
    n355 = Wait (ms)(milliseconds to wait=u32 10) -> ()  [unwired: 1 out]
    n356 = Compound Arithmetic op=OR(w547, w551) -> (w549:bool)
    n357 = control-ref of="This VI"() -> (w550:refnum<vi>)
    n358 = call "EdgeTrigger.vi"("Input Signal"=w549) -> ("Falling Edge Trigger"=w548:bool)  [unwired: 2 out]
    n359 = case shown="False" w549 {
      tunnel: w550 -> [w556 w563]
      tunnel: w548 -> [w554 _]
      frame False {
        n360 = case shown="True" w554 {
          tunnel: T21 {"Left"=100, "Top"=100, "Right"=1390, "Bottom"=585} ("Front Panel Window:Window Bounds") -> [_ w562]
          tunnel: w556 -> [w559 w561]
          tunnel: [w559 w560] -> w555
          frame False {
          }
          frame True {
            n361 = property class="VI"(reference=w561, "Front Panel.WinBounds"=w562) -> (reference out=w560:refnum<vi>)  [unwired: 1 in, 1 out]
          }
        }
        n362 = property class="VI"(reference=w555, "Front Panel.TitleBarVis"=TRUE ("Front Panel Window:Title Bar Visible")) -> ()  [unwired: 1 in, 2 out]
      }
      frame True {
        n363 = property class="VI"(reference=w563, "Front Panel.WinBounds"=T21 {"Left"=0, "Top"=0, "Right"=1290, "Bottom"=485} ("Front Panel Window:Window Bounds"), "Front Panel.TitleBarVis"=FALSE ("Front Panel Window:Title Bar Visible")) -> ()  [unwired: 1 in, 2 out]
      }
    }
  }
  n364 = while {
    tunnel: w20 -> [w569]
    tunnel: w19 -> [_]
    tunnel: w17 -> [w568]
    tunnel: w12 -> [w567]
    tunnel: w2 -> [w566]
    stop <- FALSE stop-if-true
    # "Process UI events related to test mode, checklist, and camera settings"
    n365 = event shown="[0] Timeout" {
      selector: w569 -> [_ _ _ _]
      dyn-events: _ -> [_ _ _ _]
      timeout: u32 60 ("milliseconds to wait") -> [_ _ _ _]
      tunnel: w568 -> [_ _ _ _]
      tunnel: w567 -> [_ _ _ _]
      tunnel: w566 -> [w572 _ _ _]
      event Timeout {
        (unwired) T1."Variables" ("Dashboard Tab")
        n366 = event-data() -> ()  [unwired: 1 in, 1 out]
        n367 = case shown="\"Variables\"" "Dashboard Tab" {
          tunnel: w572 -> [_ _ _]
          frame "Tune" {
          }
          frame "TeleOp", Default {
          }
          frame "Variables" {
            w577 = string[] ["CameraPublisher", "Usage", "DB"]  # Items to initially close
            n368 = First Call?() -> (First Call?: T/F=w578:bool)
            n369 = control-ref of="Tree"() -> (w579:refnum<vi>)
            n370 = Select(t=w577, s=w578, f=string[] []) -> (s? t:f=w575:string[])
            n371 = call <vilib>:"NT Read and Format Entries as Tree.vi"("Tags to  Close"=w575, "Tree Refnum"=w579) -> ()  [unwired: 8 in, 2 out]
          }
        }
        n372 = call <vilib>:"Connextion Info.vi"() -> ("Connected"=→"NT Connection":bool)  [unwired: 10 in, 1 out]
      }
      event "CheckList": Double Click {
        # "Shift clears all"
        # "Update symbols on the listbox"
        n373 = event-data() -> ("PlatMods.Shift"=w580:bool, "Row"=w582:i32)  [unwired: 1 in]
        n374 = case shown="False" w580 {
          tunnel: w582 -> [w586 _]
          tunnel: 1 -> [w585 _]
          frame False {
            n375 = property on="CheckList" class="LstBox (strict)"() -> ("Item Symbols"=w584:i32[])  [unwired: 2 in, 2 out]
            n376 = Replace Array Subset(array=w584, new element=w585, index=w586) -> (w583:i32[])
            n377 = property on="CheckList" class="LstBox (strict)"("Item Symbols"=w583) -> ()  [unwired: 2 in, 2 out]
          }
          frame True {
            w587 = 0 ("Top Row")
            n378 = property on="CheckList" class="LstBox (strict)"() -> ("Number of Rows"=w589:u32)  [unwired: 2 in, 2 out]
            n379 = Initialize Array(0, w589) -> (w588:i32[])
            n380 = property on="CheckList" class="LstBox (strict)"("Top Row"=w587, "Value"=w587, "Item Symbols"=w588) -> ()  [unwired: 2 in, 2 out]
          }
        }
      }
      event "CheckList": Key Down {
        # "Update symbols on the listbox\nLeft and right keys check and uncheck"
        n381 = event-data() -> ("VKey"=w592:T22)  [unwired: 1 in]
        n382 = case shown="\"Left\", \"Right\"" w592 {
          selector: w592 -> [w597 _]
          tunnel: eventvkey."Left" ("VKey") -> [w595 _]
          frame "Left", "Right" {
            n383 = Equal?(x=w595, y=w597) -> (x = y?=w596:bool)
            n384 = Select(t=0, s=w596, f=1) -> (s? t:f=w598:i32)
            n385 = property on="CheckList" class="LstBox (strict)"() -> ("Item Symbols"=w601:i32[])  [unwired: 2 in, 2 out]
            n386 = Replace Array Subset(array=w601, new element=w598, index="CheckList") -> (w600:i32[])
            n387 = property on="CheckList" class="LstBox (strict)"("Item Symbols"=w600) -> ()  [unwired: 2 in, 2 out]
          }
          frame Default {
          }
        }
      }
      event "Tree": Double Click {
        n388 = event-data() -> ("PlatMods"=w607:T23, "Tag"=w604:string)  [unwired: 1 in]
        n389 = Unbundle(w607) -> ("Shift"=w606:bool)  [unwired: 4 out]
        n390 = String Subset(string=w604, length (rest)=1 ("length (rest)")) -> (substring=w603:string)  [unwired: 1 in]
        n391 = Not(x=w606) -> (.not. x?=w605:bool)
        n392 = case shown="\"/\"" w603 {
          tunnel: w604 -> [_ w609]
          tunnel: w605 -> [_ w608]
          frame Default {
          }
          frame "/" {
            n393 = call <vilib>:"NT Update Persistence.vi"("Persistence"=w608, "Name"=w609) -> ()  [unwired: 9 in, 1 out]
          }
        }
      }
    }
  }
  n394 = while {
    tunnel: w3 -> [_]
    stop <- FALSE stop-if-true
    # "Maintain LimeLight connection"
    n395 = local read "Enable_Streaming_GUI"() -> (w610:bool)
    n396 = Wait (ms)(milliseconds to wait=u32 1000) -> ()  [unwired: 1 out]
    n397 = case shown="True" w610 {
      frame False {
      }
      frame True {
        w623 = "320x240 MJPEG 22 fps" ("String")
        w617 = "mjpg:http://10.42.65.11:5800"
        w622 = "/CameraPublisher/limelight/"
        # "manually configure the NT for a single LimeLight\ncamera in order to bypass WPILib's camera\nauto-detection which fails when the NTs are refreshed\nafter the code restarts on the roboRIO"
        n398 = Concatenate Strings("ip:http://", "10.42.65.11:5800" ("string")) -> (w625:string)
        n399 = Build Array(w617, w617) -> (w627:string[])
        n400 = Concatenate Strings(w622, "source") -> (w624:string)
        n401 = Concatenate Strings(w622, "description") -> (w628:string)
        n402 = Concatenate Strings(w622, "mode") -> (w629:string)
        n403 = Build Array(w623) -> (w631:string[])
        n404 = Concatenate Strings(w622, "streams") -> (w626:string)
        n405 = Concatenate Strings(w622, "modes") -> (w630:string)
        n406 = call-poly <vilib>:"NT Write Value.vi"("value"=w625, "name"=w624) -> ()  [unwired: 9 in, 1 out]
        n407 = call-poly <vilib>:"NT Write Value.vi"("value"="limelight" ("String"), "name"=w628) -> ()  [unwired: 9 in, 1 out]
        n408 = call-poly <vilib>:"NT Write Value.vi"("value"=w623, "name"=w629) -> ()  [unwired: 9 in, 1 out]
        n409 = call-poly <vilib>:"NT Write Value.vi"("value"=w627, "name"=w626) -> ()  [unwired: 9 in, 1 out]
        n410 = call-poly <vilib>:"NT Write Value.vi"("value"=w631, "name"=w630) -> ()  [unwired: 9 in, 1 out]
      }
    }
  }
  n411 = while {
    tunnel: u16 1741 ("timeout ms (25000)") -> [w633]
    stop <- FALSE stop-if-true
    # "Wait for DS connections"
    n412 = TCP Create Listener(10:w633) -> (0:w632:errorcluster, 3:w634:refnum<k5>)  [unwired: 4 in, 1 out]
    n413 = case shown="No Error" w632 {
      selector: w632 -> [w636 _]
      tunnel: w634 -> [w637 _]
      frame No Error {
        n414 = while {
          tunnel: w637 -> [w640]
          tunnel: w636 -> [w639]
          stop <- FALSE stop-if-true
          n415 = TCP Wait On Listener(8:w639, 11:w640) -> (0:w641:errorcluster, 4:w642:refnum<k5>)  [unwired: 2 in, 3 out]
          n416 = local write "TCP"(w642) -> ()
          n417 = case shown="Error" w641 {
            frame No Error {
            }
            frame Error {
              n418 = Wait (ms)(milliseconds to wait=u32 1000) -> ()  [unwired: 1 out]
            }
          }
        }
      }
      frame Error {
        n419 = Wait (ms)(milliseconds to wait=u32 1000) -> ()  [unwired: 1 out]
      }
    }
  }
  n420 = while {
    shift-right: [w656] -> _
    shift-left: _ -> [w708]
    shift-right: [w657] -> _
    shift-left: _ -> [w698]
    tunnel: w1 -> [_]
    stop <- FALSE stop-if-true
    # "Dynamic Overlays"
    n421 = To Long Integer(number="Reticule") -> (32bit integer=w689:i32)
    n422 = Wait (ms)(milliseconds to wait=u32 100) -> ()  [unwired: 1 out]
    n423 = Multiply(x=w689, y=2) -> (x*y=w688:i32)
    n424 = control-ref of="WA_Ret_Left"() -> (w670:refnum<vi>)
    n425 = control-ref of="WA_Ret_Right"() -> (w669:refnum<vi>)
    n426 = control-ref of="LL_Ret_Left"() -> (w655:refnum<vi>)
    n427 = control-ref of="LL_Ret_Right"() -> (w654:refnum<vi>)
    n428 = Increment(x=w688) -> (x+1=w676:i32)
    n429 = First Call?() -> (First Call?: T/F=w679:bool)
    n430 = Index Array(array=w698, index #1=w688, index #2=w676) -> (element #1=w692:i32, element #2=w700:i32)
    n431 = Or(x="Up", y="Down") -> (x .or. y?=w704:bool)
    n432 = Or(x="Left", y="Right") -> (x .or. y?=w694:bool)
    n433 = case shown="True" w679 {
      tunnel: [w719 w732] -> w656
      tunnel: w708 -> [w719 _]
      tunnel: w670 -> [_ w731]
      tunnel: w669 -> [_ w730]
      tunnel: w655 -> [_ w721]
      tunnel: w654 -> [_ w720]
      frame False {
      }
      frame True {
        n434 = property class="Bool (strict)"(reference=w731) -> ("Left"=w729:i32, "Top"=w728:i32)  [unwired: 1 in, 2 out]
        n435 = property class="Bool (strict)"(reference=w730) -> ("Left"=w727:i32, "Top"=w726:i32)  [unwired: 1 in, 2 out]
        n436 = property class="Bool (strict)"(reference=w721) -> ("Left"=w725:i32, "Top"=w724:i32)  [unwired: 1 in, 2 out]
        n437 = property class="Bool (strict)"(reference=w720) -> ("Left"=w723:i32, "Top"=w722:i32)  [unwired: 1 in, 2 out]
        n438 = Build Array(w729, w728, w727, w726, w725, w724, w723, w722) -> (w732:i32[])
      }
    }
    n439 = Bundle("WA_Ret_Left"=w670, "WA_Ret_Right"=w669, "LL_Ret_Left"=w655, "LL_Ret_Right"=w654) -> (w661:T24)  [unwired: 1 in]
    n440 = Decrement(x=w700) -> (x-1=w707:i32)
    n441 = Increment(x=w700) -> (x+1=w706:i32)
    n442 = Decrement(x=w692) -> (x-1=w697:i32)
    n443 = Increment(x=w692) -> (x+1=w696:i32)
    n444 = Select(t=w707, s="Up", f=w706) -> (s? t:f=w705:i32)
    n445 = Select(t=w697, s="Left", f=w696) -> (s? t:f=w695:i32)
    n446 = Select(t=w705, s=w704, f=w700) -> (s? t:f=w675:i32)
    n447 = Select(t=w695, s=w694, f=w692) -> (s? t:f=w693:i32)
    n448 = Replace Array Subset(array=w698, new element #1=w693, index #1=w688, new element #2=w675, index #2=w676) -> (w674:i32[])
    n449 = Current VI's Path() -> (path=w684:path)
    n450 = Strip Path(path=w684) -> (stripped path=w683:path)  [unwired: 1 out]
    n451 = Cluster To Array(cluster=w661) -> (array=w673:refnum<vi>[])
    n452 = Strip Path(path=w683) -> (stripped path=w645:path)  [unwired: 1 out]
    n453 = Array Size(array=w673) -> (size(s)=w672:i32)
    n454 = Build Path(base path=w645, name or relative path=path "reticule positions" ("XML File Path")) -> (appended path=w682:path)
    n455 = Multiply(x=2 ("dimension size"), y=w672) -> (x*y=w678:i32)
    n456 = Initialize Array(0, w678) -> (w668:i32[])
    n457 = call-poly <vilib>:"Read From XML File.vi"("XML File Path"=w682) -> ("error out"=w660:errorcluster, "XML Elements"=w681:string[])  [unwired: 8 in, 1 out]
    n458 = case shown="No Error" w660 {
      tunnel: w681 -> [w715 _]
      tunnel: w668 -> [w712 _]
      tunnel: [w711 i32[] [0, 0, 0, 0, 0, 0, 0, 0, 0, 0, 0, 0] ("value")] -> w658
      frame No Error {
        n459 = Index Array(array=w715, index=0) -> (element=w713:string)
        n460 = Unflatten From XML(xml string=w713, type=w712) -> (value=w711:i32[])  [unwired: 1 in, 1 out]
      }
      frame Error {
      }
    }
    n461 = First Call?() -> (First Call?: T/F=w699:bool)
    n462 = Select(t=w658, s=w699, f=w674) -> (s? t:f=w657:i32[])
    n463 = Add(x=w657, y=w656) -> (x+y=w659:i32[])
    n464 = Index Array(array=w659, index #1=0 ("index")) -> (element #1=w665:i32, element #2=w664:i32, element #3=w663:i32, element #4=w662:i32, element #5=w653:i32, element #6=w652:i32, element #7=w651:i32, element #8=w650:i32)  [unwired: 7 in]
    n465 = Unbundle(w661) -> ("WA_Ret_Left"=w666:refnum<vi>, "WA_Ret_Right"=w667:refnum<vi>, "LL_Ret_Left"=w649:refnum<vi>, "LL_Ret_Right"=w648:refnum<vi>)
    n466 = Flatten To XML(6:w657) -> (2:w686:string)
    n467 = call "EdgeTrigger.vi"("Input Signal"="Save") -> ("Rising Edge Trigger"=w646:bool)  [unwired: 2 out]
    n468 = case shown="True" w646 {
      tunnel: w686 -> [_ w718]
      tunnel: w682 -> [_ w717]
      frame False {
      }
      frame True {
        n469 = call-poly <vilib>:"Write to XML File.vi"("XML Input"=w718, "XML File Path"=w717) -> ()  [unwired: 7 in, 3 out]
      }
    }
    n470 = property class="Bool (strict)"(reference=w666, "Left"=w665, "Top"=w664) -> ()  [unwired: 1 in, 2 out]
    n471 = property class="Bool (strict)"(reference=w667, "Left"=w663, "Top"=w662) -> ()  [unwired: 1 in, 2 out]
    n472 = property class="Bool (strict)"(reference=w649, "Left"=w653, "Top"=w652) -> ()  [unwired: 1 in, 2 out]
    n473 = property class="Bool (strict)"(reference=w648, "Left"=w651, "Top"=w650) -> ()  [unwired: 1 in, 2 out]
  }
  n474 = while {
    tunnel: w10 -> [w762]
    tunnel: w3 -> [w746]
    tunnel: w4 -> [w744]
    stop <- FALSE stop-if-true
    w733 = u16 0 items=["Stop", "Record", "Playback Panel"] ("Rec Mode")
    # "Camera Feeds"
    n475 = First Call?() -> (First Call?: T/F=w740:bool)
    n476 = local read "NT Connection"() -> (w743:bool)
    n477 = call "Timer.vi"("Reset Timer"=w740) -> ("Time (ms)"=w739:u32)
    n478 = Greater?(x=w739, y=u32 5000) -> (0:w737:bool)
    n479 = Compound Arithmetic op=AND(w743, "Enable_Streaming_GUI", w737) -> (w742:bool)
    n480 = Bundle("Camera Name"="Camera Name", w746, "Saved DB Images Info"=w762) -> (w761:T25)  [unwired: 1 in]
    n481 = control-ref of="Camera Perf"() -> (w759:refnum<vi>)
    n482 = call <vilib>:"WPI_CameraRead MJPG for Dashboard_2.vi"("Camera Settings"="Camera Settings", "Rec Mode"=w733, "NT Connection"=w742, "Capture Info"=w761, "Image in"=w744) -> ("perf info"=w760:cluster{"Bandwidth (Mbps)":dbl, "fps":dbl}, "Active"=w745:bool, "Image\\ out"=w763:T3)  [unwired: 4 in]
    n483 = call <vilib>:"WPI_DashboardFormatPerf.vi"("Right Camera Perf"=cluster{"Bandwidth (Mbps)":dbl, "FPS":dbl} {"Bandwidth (Mbps)"=0.0, "FPS"=0.0}, "Performance"=w760, "String in"=w759) -> ()  [unwired: 9 in]
    n484 = case shown="True" w745 {
      tunnel: w763 -> [w774 w777]
      tunnel: [w774 w776] -> w758
      frame False {
        n485 = Wait Until Next ms Multiple(millisecond multiple=u32 500) -> ()  [unwired: 1 out]
      }
      frame True {
        # "image annotation etc."
        n486 = call "IMAQ Clear Overlay"("Image"=w777) -> ("Image Out"=w776:T3)  [unwired: 2 in, 8 out]
      }
    }
    n487 = call "IMAQ Rotate"("Angle (degrees)"=sgl 0.0, "Image Src"=w758) -> ("Image Dst Out"=w749:T3)  [unwired: 8 in, 1 out]
    n488 = call "IMAQ GetImageSize"("Image"=w749) -> ("Y Resolution"=w747:i32, "X Resolution"=w734:i32)  [unwired: 3 in, 1 out]
    n489 = To Double Precision Float(number=w734) -> (double precision float=w756:dbl)
    n490 = To Double Precision Float(number=w747) -> (double precision float=w755:dbl)
    n491 = Divide(x=w756, y=w755) -> (x/y=w754:dbl)
    n492 = Less?(x=w754, y=1.9) -> (x < y?=→"No_Secondary_Camera":bool)
    n493 = case shown="160, Default" w734 {
      tunnel: "Partial Video Stream" ("Image Name") -> [_ w773]
      tunnel: [w765 w772] -> w736
      tunnel: w749 -> [w765 w770]
      frame 320 {
        # "wide angle camera found"
      }
      frame 160, Default {
        w766 = T11 4 items=["Grayscale (U8)", "Grayscale (I16)", "Grayscale (SGL)", "Complex (CSG)", "RGB (U32)", "HSL (U32)", "RGB (U64)"] ("Image Type")
        # "no wide angle camera found"
        n494 = call "IMAQ Create"("Image Name"=w773, "Image Type"=w766) -> ("New Image"=w769:T3)  [unwired: 3 in, 1 out]
        n495 = call "IMAQ SetImageSize"("Y Resolution"=120, "X Resolution"=320, "Image"=w769) -> ("Image Out"=w771:T3)  [unwired: 2 in, 1 out]
        n496 = call "IMAQ ImageToImage 2"("Image Src (Small)"=w770, "Image Src (Large)"=w771) -> ("Image Dst Out"=w772:T3)  [unwired: 8 in, 1 out]
      }
    }
    "Combined Camera Feed" <- w736
  }
  n497 = while {
    stop <- FALSE stop-if-true
    # "Error Message Handling"
    n498 = property on="Actuator Testing" class="Ring (strict)"() -> ("RingText.Text"=w815:string)  [unwired: 2 in, 2 out]
    n499 = local read "Master_Safety_Override_1"() -> (w786:bool)
    n500 = local read "Arm_Calibrate_Wheels_GUI"() -> (w835:bool)
    n501 = local read "Arm_Calibrate_Joysticks"() -> (w805:bool)
    n502 = local read "Swerve_Shifter_Failure"() -> (w796:bool)
    n503 = local read "CAN_Bus_Fault_GUI"() -> (w802:bool)
    n504 = Wait (ms)(milliseconds to wait=u32 200) -> ()  [unwired: 1 out]
    n505 = local read "Swerve_Azimuth_Fault"() -> (w839:bool)
    n506 = Not Equal?(x=w815, y="No_Test") -> (x != y?=w822:bool)
    n507 = local read "Home_Wheels_GUI"() -> (w788:bool)
    n508 = local read "Swerve_Overheating"() -> (w848:bool)
    n509 = local read "Super_Test_Mode_GUI"() -> (w856:bool)
    n510 = call <vilib>:"Space Constant.vi"() -> ("String"=w813:string)
    n511 = local read "Swerve_Drive_Fault"() -> (w779:bool)
    n512 = local read "Auto_Test_Mode_GUI"() -> (w827:bool)
    n513 = local read "IMU_Failure_GUI"() -> (w819:bool)
    n514 = local read "Electrical_Fault_GUI"() -> (w810:bool)
    n515 = local read "Vision_Fault_GUI"() -> (w783:bool)
    n516 = local read "Pressure_Vent_GUI"() -> (w844:bool)
    n517 = local read "Auto_Error_GUI"() -> (w832:bool)
    n518 = Search and Replace String(replace all?=TRUE ("replace all? (F)"), input string=w815, search string="_", replace string=w813) -> (result string=w816:string)  [unwired: 4 in, 3 out]
    n519 = local read "Slow_Loop"() -> (w851:bool)
    n520 = Concatenate Strings("testing " ("string"), w816) -> (w825:string)
    n521 = Bundle("homing the wheels", "Home_Wheels_GUI"=w788, 60.0) -> (w787:cluster{string, "Home_Wheels_GUI":bool, dbl})  [unwired: 1 in]
    n522 = Bundle("swerve shifter failure, forced into low gear", "Swerve_Shifter_Failure"=w796, 600.0) -> (w795:T26)  [unwired: 1 in]
    n523 = Bundle("Lime Light failure", "Vision_Fault_GUI"=w783, 600.0) -> (w782:cluster{string, "Vision_Fault_GUI":bool, dbl})  [unwired: 1 in]
    n524 = Bundle("swerve drive failure", "Swerve_Drive_Fault"=w779, 600.0) -> (w778:cluster{string, "Swerve_Drive_Fault":bool, dbl})  [unwired: 1 in]
    n525 = Bundle("safeties disengaged", "Master_Safety_Override_1"=w786, 10.0) -> (w860:T27)  [unwired: 1 in]
    n526 = Bundle("disabled test mode", "Super_Test_Mode_GUI"=w856, 10.0) -> (w859:cluster{string, "Super_Test_Mode_GUI":bool, dbl})  [unwired: 1 in]
    n527 = Bundle("control latency too high", "Slow_Loop"=w851, 60.0) -> (w852:cluster{string, "Slow_Loop":bool, dbl})  [unwired: 1 in]
    n528 = Bundle("drive train overheating", "Swerve_Overheating"=w848, 60.0) -> (w847:cluster{string, "Swerve_Overheating":bool, dbl})  [unwired: 1 in]
    n529 = Bundle("pressure venting", "Pressure_Vent_GUI"=w844, 600.0) -> (w843:cluster{string, "Pressure_Vent_GUI":bool, dbl})  [unwired: 1 in]
    n530 = Bundle("swerve azimuth failure", "Swerve_Azimuth_Fault"=w839, 600.0) -> (w840:T28)  [unwired: 1 in]
    n531 = Bundle("ready to calibrate swerve modules", "Arm_Calibrate_Wheels_GUI"=w835, 10.0) -> (w836:T29)  [unwired: 1 in]
    n532 = Bundle("autonomous play failure", "Auto_Error_GUI"=w832, 10.0) -> (w831:cluster{string, "Auto_Error_GUI":bool, dbl})  [unwired: 1 in]
    n533 = Bundle("autonomous test mode", "Auto_Test_Mode_GUI"=w827, 10.0) -> (w828:cluster{string, "Auto_Test_Mode_GUI":bool, dbl})  [unwired: 1 in]
    n534 = Bundle(w825, w822, 10.0) -> (w821:cluster{string, bool, dbl})  [unwired: 1 in]
    n535 = Bundle("IMU failure, auto-targeting disabled", "IMU_Failure_GUI"=w819, 600.0) -> (w817:cluster{string, "IMU_Failure_GUI":bool, dbl})  [unwired: 1 in]
    n536 = Bundle("electrical bus fault, power down", "Electrical_Fault_GUI"=w810, 60.0) -> (w809:T30)  [unwired: 1 in]
    n537 = Bundle("ready to calibrate joysticks, wait ten seconds after pressing calibrate", "Arm_Calibrate_Joysticks"=w805, 10.0) -> (w806:T31)  [unwired: 1 in]
    n538 = Bundle("CAN bus fault, check wiring", "CAN_Bus_Fault_GUI"=w802, 60.0) -> (w804:cluster{string, "CAN_Bus_Fault_GUI":bool, dbl})  [unwired: 1 in]
    n539 = local read "Audible_Warnings_Enabled_GUI"() -> (w794:bool)
    n540 = Build Array(w860, w859, w852, w847, w843, w840, w836, w831, w828, w821, w817, w809, w806, w804, w795, w787, w782, w778) -> (w858:T32)
    n541 = call "EdgeTrigger.vi"("Input Signal"=w794) -> ("All Edge Trigger"=w793:bool)  [unwired: 2 out]
    n542 = call "ErrorMessageBuilder.vi"("Errors"=w858, "Reset Error History"=w793) -> ("Combined Error String"=w799:string)
    n543 = Not Equal?(x="", y=w799) -> (x != y?=w800:bool)
    n544 = Compound Arithmetic op=AND(w794, w800) -> (w792:bool)
    n545 = case shown="True" w792 {
      tunnel: w799 -> [_ w867]
      frame False {
      }
      frame True {
        n546 = call "TextToSpeech.vi"("Text To Be Spoken"=w867) -> ()  [unwired: 9 in, 2 out]
      }
    }
    n547 = case shown="True" w800 {
      tunnel: w799 -> [_ w866]
      frame False {
      }
      frame True {
        "Combined Error String" <- w866
      }
    }
  }
